vi "LV to ITX  Retrieve_SE mode.vi"(0 "File or Folder Path":path=path "G:/My Drive/ansom/Data/PPMS2/SA03008L.20190612/030_phi_90_Vamp_bg=30_IV_Testing/SA03008L.20190612.000014.itx", 5 "offset":i32, 7 "length":i32=1, 9 "index":T2={"A"=7, "B"=17, "C"=7, "D"=17, "E"=3, "N1"=2, "N2"=2, "N3"=3, "N4"=4, "A 1"=3, "A 2"=3, "C 1"=3, "C 2"=3, "E 2"=4}, 11 "stop":bool, 12 "file contains 2D data?":bool) -> (1 "Spherical coordinates":dbl[][](array[numeric]), 2 "long":cluster{i32[], dbl[]}(graph), 3 "G vs T":cluster{dbl[], dbl[]}(graph), 4 "A vs B":cluster{dbl[], dbl[]}[](graph), 6 "C vs D":cluster{dbl[], dbl[]}[](graph), 8 "E( = A)":dbl[][](graph)=[[1.0203117914485766e-05], [1.0451409415651452e-05], [1.0462825682376084e-05], [1.0239799983652948e-05], [9.906027918537444e-06], [9.668588795449023e-06], [9.554840000855235e-06], [9.476205145075346e-06], [9.320844077203883e-06], [9.198217260011043e-06], [9.317043476919502e-06], [9.695411083534662e-06], [1.0241945945024096e-05], [1.0795271186317606e-05], [1.1298338561231194e-05], [1.1790485816338598e-05], [1.2350446475265752e-05], [1.2919662467720538e-05], [1.3290994889745302e-05], [1.3411667855331416e-05], [1.330535085371591e-05], [1.3128995145360939e-05], [1.3030460580636378e-05], [1.2978894707939279e-05], [1.2876874119941293e-05], [1.2686944824355687e-05], [1.2580403309284722e-05], [1.2658289461507464e-05], [1.2907014184352959e-05], [1.3250891765203631e-05], [1.3571060207080296e-05], [1.38696075611843e-05], [1.4181218154607563e-05], [1.4550968177813745e-05], [1.4864220110273978e-05], [1.4963626262998592e-05], [1.483786218451115e-05], [1.454789392231275e-05], [1.4276013976759574e-05], [1.4093434987113507e-05], [1.394115331370823e-05], [1.3733942398008014e-05], [1.3498551722113728e-05], [1.3401834118376352e-05], [1.349625299977089e-05], [1.376633995345719e-05], [1.4099700190262174e-05], [1.439564212454811e-05], [1.4669263029595617e-05], [1.4993648567227242e-05], [1.5385015866889246e-05], [1.564851404848794e-05], [1.5665209617742956e-05], [1.5433872809106696e-05], [1.5053460371993616e-05], [1.4698589553022668e-05], [1.4387375425877016e-05], [1.4045380848753723e-05], [1.3602477208659444e-05], [1.3177214908981591e-05], [1.2924329669653593e-05], [1.2880547914446448e-05], [1.303231603971595e-05], [1.3248510272418485e-05], [1.3465963014008446e-05], [1.3681644430620408e-05], [1.3944747365597995e-05], [1.4215309953351151e-05], [1.431037322959714e-05], [1.4175945939035027e-05], [1.3817874591680678e-05], [1.3391248811154445e-05], [1.3062055548545288e-05], [1.2821830137320284e-05], [1.2576309609254846e-05], [1.2246815447133818e-05], [1.1922180751465795e-05], [1.1680853926483689e-05], [1.1589134778894471e-05], [1.1633830542786138e-05], [1.1704064673099467e-05], [1.1789993030575904e-05], [1.1926922111402669e-05], [1.215771870713351e-05], [1.2337490622128459e-05], [1.230294631547821e-05], [1.2038499839080447e-05], [1.1589020929183376e-05], [1.1155486186825546e-05], [1.0841489539352708e-05], [1.0586914588993357e-05], [1.0275705901404508e-05], [9.933726372538684e-06], [9.741201124246198e-06], [9.759761104382419e-06], [9.991224895934066e-06], [1.0316901386610578e-05], [1.0633212529286809e-05], [1.0935414635607847e-05], [1.127192689353356e-05], [1.168222121368369e-05], [1.1975070483694205e-05], [1.2017866014802864e-05], [1.182059565925867e-05], [1.1495227673116619e-05], [1.1221973090195048e-05], [1.102061719762733e-05], [1.0822809552516617e-05], [1.0531987977837665e-05], [1.0230877354511187e-05], [1.0096596104104945e-05], [1.0173052237292175e-05], [1.0421846888649233e-05], [1.0702637025924256e-05], [1.095426977171788e-05], [1.1200388597928466e-05], [1.1519306746724885e-05], [1.1877703630116518e-05], [1.2078276877349205e-05], [1.205320354878895e-05], [1.1810154186171108e-05], [1.1490160906859651e-05], [1.1235411490808346e-05], [1.1028963796796881e-05], [1.0777926144571402e-05], [1.0435400507185421e-05], [1.0169646968721249e-05], [1.010128110333465e-05], [1.0231121727379654e-05], [1.0469283566468044e-05], [1.0678876882796116e-05], [1.0845441918195888e-05], [1.1013496058458993e-05], [1.1250653310333545e-05], [1.1455840654342756e-05], [1.1487198402341834e-05], [1.1316332482261583e-05], [1.0965676444491303e-05], [1.0604440631932836e-05], [1.0327624088147793e-05], [1.0096830398805317e-05], [9.811227194429744e-06], [9.511062174305784e-06], [9.433820234221822e-06], [9.65222061750109e-06], [1.0092082217056494e-05], [1.0586760382445729e-05], [1.101426996619165e-05], [1.1384440045107256e-05], [1.1767057215702233e-05], [1.218251607479168e-05], [1.245159787228818e-05], [1.2481102402364999e-05], [1.2291430480708847e-05], [1.1986335326318682e-05], [1.1733869529760309e-05], [1.1548603391828037e-05], [1.13596762158455e-05], [1.1087736184421201e-05], [1.0839800019004791e-05], [1.076298217931536e-05], [1.087176289143856e-05], [1.1137984996962431e-05], [1.142759878667849e-05], [1.1672564147584565e-05], [1.189430562660553e-05], [1.2172128947557167e-05], [1.2459795985893852e-05], [1.2561260005336956e-05], [1.2424412782407364e-05], [1.2054150550705076e-05], [1.1589880038662732e-05], [1.1192416052986661e-05], [1.0863456381263106e-05], [1.051505112264767e-05], [1.0100597815099605e-05], [9.761572319705686e-06], [9.570513017820516e-06], [9.543303173198097e-06], [9.642325412517067e-06], [9.74774836365151e-06], [9.858949953493099e-06], [1.001903548052811e-05], [1.0256078261757475e-05], [1.0439598776211572e-05], [1.042242238004522e-05], [1.0183216760688765e-05], [9.769220768503082e-06], [9.367514440383908e-06], [9.053677195274377e-06], [8.770462725955242e-06], [8.43425116077764e-06], [8.081231920036751e-06], [7.879765327297044e-06], [7.889913212940979e-06], [8.1260164848618e-06], [8.447281143591908e-06], [8.695609460809765e-06], [8.902012120386912e-06], [9.171053878914142e-06], [9.519041688511399e-06], [9.760420847561693e-06], [9.77389276916549e-06], [9.538471022579816e-06], [9.15889899491702e-06], [8.826822020269094e-06], [8.565524931184424e-06], [8.289350815712172e-06], [7.8969407152003e-06], [7.459738307347468e-06], [7.128929719791946e-06], [6.99557875543524e-06], [7.060672622112839e-06], [7.158874263853444e-06], [7.221292908402365e-06], [7.283320382366653e-06], [7.412810700573441e-06], [7.557741133867653e-06], [7.536052902423093e-06], [7.301346793160131e-06], [6.860798082904608e-06], [6.352981206582646e-06], [5.915198962346519e-06], [5.513485928879271e-06], [5.042056071494383e-06], [4.47272121028262e-06], [3.990706674059657e-06], [3.711277759527869e-06], [3.648286875837285e-06], [3.736276427208576e-06], [3.846408121208589e-06], [3.94839189517527e-06], [4.081067676347965e-06], [4.321202984988554e-06], [4.539701763689317e-06], [4.560691591500203e-06], [4.362959065752805e-06], [4.00747885911292e-06], [3.684539738102325e-06], [3.457908230535235e-06], [3.256577421797549e-06], [2.982077739421097e-06], [2.677707243957301e-06], [2.527995181945928e-06], [2.563590932568395e-06], [2.757244015651364e-06], [3.004506737628388e-06], [3.216838705464376e-06], [3.411720821800805e-06], [3.65592557254819e-06], [3.966380574944244e-06], [4.154977498960543e-06], [4.109249917249561e-06], [3.827641578709879e-06], [3.415103581151261e-06], [3.060145017851194e-06], [2.788449265930315e-06], [2.531428415712389e-06], [2.223813484173366e-06], [1.961951236414797e-06], [1.873175358972362e-06], [1.978752723280979e-06], [2.235548987483699e-06], [2.487500911952594e-06], [2.680258099595024e-06], [2.857726048616139e-06], [3.101374069773001e-06], [3.360530904168342e-06], [3.439879860822285e-06], [3.285712948159889e-06], [2.920853244361546e-06], [2.517085401731428e-06], [2.227960344817152e-06], [2.019360394093301e-06], [1.790712123384404e-06], [1.490453406785682e-06], [1.314481541186986e-06], [1.436226320267349e-06], [1.830555611405548e-06], [2.347376474778584e-06], [2.83276224941652e-06], [3.273270977299852e-06], [3.720804122713015e-06], [4.225387814657854e-06], [4.643762651590139e-06], [4.818501878615677e-06], [4.74287964664764e-06], [4.484016645670352e-06], [4.23197417456386e-06], [4.052188441737428e-06], [3.878583078383493e-06], [3.6213318980411e-06], [3.320427547442246e-06], [3.144570932206806e-06], [3.145190133720137e-06], [3.342213788958479e-06], [3.643982192034937e-06], [3.950314414020666e-06], [4.273802952804333e-06], [4.665541321937886e-06], [5.116145221529651e-06], [5.437284100346412e-06], [5.532627391374035e-06], [5.39754437705853e-06], [5.128169611859323e-06], [4.896411012736348e-06], [4.725729377989505e-06], [4.570373201814337e-06], [4.358936049799571e-06], [4.191322167244521e-06], [4.217144518716558e-06], [4.445677705144123e-06], [4.827234705535528e-06], [5.222470576927392e-06], [5.582610826085262e-06], [5.934955025393205e-06], [6.340159015530785e-06], [6.731834383113837e-06], [6.909189589337826e-06], [6.827526507809335e-06], [6.512808994630573e-06], [6.124039292062173e-06], [5.789316724794161e-06], [5.474577386936262e-06], [5.115423045986515e-06], [4.695085634491939e-06], [4.371814745650077e-06], [4.238329052844964e-06], [4.29836974160633e-06], [4.47838263827086e-06], [4.6479008090333e-06], [4.787126253382991e-06], [4.932759271760401e-06], [5.15222285566227e-06], [5.314443835593722e-06], [5.249888099863707e-06], [4.955396042759312e-06], [4.49094662616732e-06], [4.032573470572639e-06], [3.652538610621264e-06], [3.289848568538427e-06], [2.862668862863305e-06], [2.386109658112519e-06], [1.980877493646386e-06], [1.723813276391883e-06], [1.666466791653346e-06], [1.708598627200872e-06], [1.750958161424472e-06], [1.803408641811402e-06], [1.924580144024447e-06], [2.131889646664636e-06], [2.23190345117017e-06], [2.101992507805945e-06], [1.746313784890978e-06], [1.282165699648718e-06], [9.008654645192786e-07], [6.245874645948886e-07], [3.603328178056157e-07], [1.2850462096549098e-08], [-2.9789678292108053e-07], [-3.9750583982440066e-07], [-2.555823624812689e-07], [7.11177067009668e-08], [4.2320008921387924e-07], [7.487434826133602e-07], [1.066972084992825e-06], [1.434819215080255e-06], [1.800878646893036e-06], [1.959611245457595e-06], [1.853971362801683e-06], [1.516878911187727e-06], [1.117968181486286e-06], [7.985815688218983e-07], [5.096106220425769e-07], [1.4977550826058187e-07], [-2.946925906959275e-07], [-6.300191196025e-07], [-7.439538241958556e-07], [-6.359796849249192e-07], [-3.886910298714256e-07], [-1.3897634048540907e-07], [9.549038154863474e-08], [3.508743558744578e-07], [6.84545669886253e-07], [9.691078084455289e-07], [1.045482439389716e-06], [8.974995121583454e-07], [5.802282921684991e-07], [2.7770754230560435e-07], [6.055233896067443e-08], [-1.217629251957688e-07], [-3.541677543525877e-07], [-5.957703521256667e-07], [-6.864721271250091e-07], [-5.986966950738157e-07], [-3.3156894730776936e-07], [-2.272892874096102e-09], [2.6674322548996125e-07], [4.88776088221634e-07], [7.363185836564282e-07], [1.030874484092974e-06], [1.204371480070388e-06], [1.161248106198924e-06], [8.881766431856405e-07], [4.88182629381204e-07], [1.6957924160034613e-07], [-3.531580448202741e-08], [-1.997832893026395e-07], [-4.102211628754495e-07], [-5.710429951959878e-07], [-4.961172001967793e-07], [-1.5114185155885382e-07], [3.744481859043512e-07], [9.191159334167871e-07], [1.430499110631943e-06], [1.919253087931085e-06], [2.445675439460715e-06], [2.988121323760386e-06], [3.368179636685896e-06], [3.48351381168019e-06], [3.322399885005343e-06], [3.07056014534199e-06], [2.903753127818985e-06], [2.79632673000765e-06], [2.637584615085359e-06], [2.383878891964776e-06], [2.203073403682545e-06], [2.206283438080234e-06], [2.405450646883647e-06], [2.716423840938837e-06], [2.997254703288021e-06], [3.241467706370339e-06], [3.511794372749976e-06], [3.868311613144331e-06], [4.15533629381371e-06], [4.203690567256924e-06], [4.006419102954573e-06], [3.618876334099121e-06], [3.236053706440711e-06], [2.934280935773519e-06], [2.643883040603065e-06], [2.264492261057744e-06], [1.851511625129745e-06], [1.612134189405098e-06], [1.583215981848726e-06], [1.729201609841909e-06], [1.944355531860828e-06], [2.13024641884391e-06], [2.283816621994958e-06], [2.477461369183668e-06], [2.728587070825201e-06], [2.847811614538933e-06], [2.751491004377477e-06], [2.449412680323661e-06], [2.044435640440341e-06], [1.721446280484857e-06], [1.497770951345898e-06], [1.293161644964387e-06], [1.010439134397641e-06], [7.454181515776826e-07], [6.603433933302327e-07], [7.876365575969897e-07], [1.086288853957634e-06], [1.410545885540973e-06], [1.70814523635708e-06], [2.018512138600734e-06], [2.421154123964878e-06], [2.851042034185028e-06], [3.09276890545274e-06], [3.091227660951088e-06], [2.872414028807718e-06], [2.596154472420182e-06], [2.405449023316103e-06], [2.274691555343845e-06], [2.10839650320063e-06], [1.8405205006478e-06], [1.588796015095602e-06], [1.460207742292944e-06], [1.516317184332083e-06], [1.712469405531179e-06], [1.901116704222114e-06], [2.050382524275238e-06], [2.208421297738088e-06], [2.444117414591197e-06], [2.646666143304353e-06], [2.668691134184238e-06], [2.474176299410271e-06], [2.105949975915483e-06], [1.765464179910295e-06], [1.526397172225546e-06], [1.32946264448765e-06], [1.088560883676088e-06], [8.227278560205486e-07], [6.864402022873568e-07], [7.299174399197152e-07], [9.672335319015463e-07], [1.30141719424543e-06], [1.6208334069415e-06], [1.913529408708613e-06], [2.220449994366263e-06], [2.563869674397319e-06], [2.788889776922702e-06], [2.791337202094483e-06], [2.559998735141068e-06], [2.201772202390378e-06], [1.899596496537296e-06], [1.672853353150462e-06], [1.444512065193071e-06], [1.128819750981524e-06], [8.408771228283138e-07], [7.573676174365871e-07], [9.045652354797287e-07], [1.222661558811304e-06], [1.572171244126944e-06], [1.892799603038695e-06], [2.194159561400824e-06], [2.55808916828674e-06], [2.929781042095453e-06], [3.105640547296532e-06], [3.04470953591822e-06], [2.77985109235159e-06], [2.477765739299556e-06], [2.263806449175554e-06], [2.089337566626353e-06], [1.857038796143934e-06], [1.531643873879591e-06], [1.287254079771486e-06], [1.228018805637217e-06], [1.359929120505531e-06], [1.626954183030257e-06], [1.899503641261853e-06], [2.149083748605454e-06], [2.424318021443189e-06], [2.771058966258793e-06], [3.03779347608129e-06], [3.070950972178974e-06], [2.862310179591683e-06], [2.472534202116903e-06], [2.08701427800541e-06], [1.773191081900734e-06], [1.475834316236762e-06], [1.107346170237545e-06], [7.217834878283793e-07], [5.400379788174451e-07], [6.384864116813995e-07], [9.723852081279428e-07], [1.394457283972456e-06], [1.800063013342451e-06], [2.192915874449245e-06], [2.620621076879388e-06], [3.089354051541878e-06], [3.43075078848014e-06], [3.535509574751654e-06], [3.385605436421143e-06], [3.09990916505182e-06], [2.854328439744856e-06], [2.649265060027011e-06], [2.427348435903839e-06], [2.130950149691371e-06], [1.874965331750264e-06], [1.800585266108255e-06], [1.922778247879644e-06], [2.209874864767858e-06], [2.517069382566403e-06], [2.777710512520955e-06], [3.025077599580109e-06], [3.344371123008913e-06], [3.670968838980564e-06], [3.805153528635349e-06], [3.719045967382481e-06], [3.4453056065883e-06], [3.121717158538113e-06], [2.867202531810868e-06], [2.666060001059221e-06], [2.446064840422678e-06], [2.182870825013239e-06], [2.031393827881757e-06], [2.064437873244976e-06], [2.274629467551607e-06], [2.572929205865769e-06], [2.828532692006165e-06], [3.046953258646045e-06], [3.282485366653173e-06], [3.602584247405248e-06], [3.880581588153572e-06], [3.958501824259167e-06], [3.812998042220891e-06], [3.500154747796919e-06], [3.220209945487412e-06], [3.033425363641895e-06], [2.860399775395278e-06], [2.61920739403021e-06], [2.370543731049188e-06], [2.287136477362237e-06], [2.413618613599854e-06], [2.747229106812454e-06], [3.159624133634061e-06], [3.537454804057392e-06], [3.886505667804312e-06], [4.274535372370747e-06], [4.730559591923031e-06], [5.063492431218344e-06], [5.157257415055617e-06], [5.005731444161624e-06], [4.719943355378965e-06], [4.487458764381221e-06], [4.335606809240858e-06], [4.196104531728331e-06], [3.967290069039871e-06], [3.728240982089026e-06], [3.615701464454324e-06], [3.683976766834997e-06], [3.934564789475532e-06], [4.228261965097601e-06], [4.502387528544013e-06], [4.779542484424882e-06], [5.117289121815712e-06], [5.449335107903793e-06], [5.58701981163888e-06], [5.487694869509108e-06], [5.176018183753834e-06], [4.819191726850881e-06], [4.546511619318568e-06], [4.300821328369082e-06], [3.99781338085952e-06], [3.62673275657825e-06], [3.355487904966211e-06], [3.274086263472789e-06], [3.372249691405775e-06], [3.582345894870657e-06], [3.784449257833265e-06], [3.961951546871228e-06], [4.174250564645887e-06], [4.484714742695696e-06], [4.74020001227765e-06], [4.763433680211768e-06], [4.540563757421029e-06], [4.145600443100241e-06], [3.768598878927397e-06], [3.471172633634845e-06], [3.191447933683471e-06], [2.837239398545553e-06], [2.463511586571342e-06], [2.270735427476304e-06], [2.294716771548237e-06], [2.504898408993516e-06], [2.794306132286138e-06], [3.068322981631204e-06], [3.339437133022253e-06], [3.666058584241702e-06], [4.035431693880267e-06], [4.263965590990658e-06], [4.269395932914149e-06], [4.052437885411495e-06], [3.725874661453007e-06], [3.469667161741944e-06], [3.285674775833183e-06], [3.093631254341317e-06], [2.835403027320849e-06], [2.661288889179454e-06], [2.71963741334409e-06], [2.983483155818505e-06], [3.371429906272921e-06], [3.735029322161288e-06], [4.042427897309145e-06], [4.339621134221055e-06], [4.698433044568193e-06], [5.051264781404729e-06], [5.207905217871494e-06], [5.134693036873634e-06], [4.855329659996543e-06], [4.522835077294536e-06], [4.264599217223204e-06], [4.0509608926548e-06], [3.797881884872371e-06], [3.480006869288144e-06], [3.307000859045598e-06], [3.434613753073963e-06], [3.830250793698165e-06], [4.335369985352999e-06], [4.806810326506096e-06], [5.243588355373231e-06], [5.698033177926932e-06], [6.234766917863396e-06], [6.720371003428815e-06], [6.998847270190049e-06], [7.044838590512829e-06], [6.902368063818684e-06], [6.7543073980886e-06], [6.672453056620447e-06], [6.606293176564262e-06], [6.474473183251771e-06], [6.31277456486036e-06], [6.286562865011889e-06], [6.452152101869052e-06], [6.800158649510438e-06], [7.203929198104126e-06], [7.562895282031667e-06], [7.888021258620359e-06], [8.239039473020091e-06], [8.626346460217915e-06], [8.877160655531826e-06], [8.885615965537383e-06], [8.625705887098092e-06], [8.212255192644841e-06], [7.839117684774636e-06], [7.518591920880371e-06], [7.184310792842499e-06], [6.77147094972243e-06], [6.390127428925089e-06], [6.171984080464439e-06], [6.146261082580145e-06], [6.297407503219818e-06], [6.472742201385194e-06], [6.608435299039607e-06], [6.756133415743732e-06], [7.015040583179219e-06], [7.330421268770488e-06], [7.478904508054431e-06], [7.374191363904208e-06], [7.027486025784916e-06], [6.611420746799494e-06], [6.267509783907579e-06], [5.953916635800534e-06], [5.576336008604536e-06], [5.122155234699542e-06], [4.758469980040258e-06], [4.568062244936127e-06], [4.569931379995312e-06], [4.705877665972491e-06], [4.839700599305497e-06], [4.959180515709513e-06], [5.131680469570321e-06], [5.410800967050358e-06], [5.63492714528286e-06], [5.642076968352041e-06], [5.408862788679098e-06], [4.970633871102984e-06], [4.502316899450866e-06], [4.084806234015227e-06], [3.682560840105224e-06], [3.217313239532915e-06], [2.721284890287605e-06], [2.344087479039076e-06], [2.153751782753977e-06], [2.175351195881462e-06], [2.298085624890723e-06], [2.430663518050305e-06], [2.589303835716231e-06], [2.846831744546804e-06], [3.214272130879574e-06], [3.486804163039535e-06], [3.532579461969519e-06], [3.333988553624396e-06], [3.019823207071486e-06], [2.786031977279591e-06], [2.631151717042815e-06], [2.475234004435696e-06], [2.254818436661476e-06], [2.067389328034075e-06], [2.065265302354666e-06], [2.278140295990367e-06], [2.629202221216723e-06], [2.968695184526776e-06], [3.259532435891047e-06], [3.543640533579852e-06], [3.906058832181727e-06], [4.290718558291195e-06], [4.502467158663368e-06], [4.476075533965759e-06], [4.229861183612979e-06], [3.942382521675467e-06], [3.747008475433462e-06], [3.592273249341639e-06], [3.391937829252852e-06], [3.137281734593259e-06], [2.987944717267124e-06], [3.027807941274348e-06], [3.263532901865624e-06], [3.615503595071192e-06], [3.957905863806523e-06], [4.300800643533351e-06], [4.696553717671453e-06], [5.180948646265811e-06], [5.615737328280651e-06], [5.839855918335066e-06], [5.800711875450168e-06], [5.558479023553354e-06], [5.336680797054845e-06], [5.21988745057688e-06], [5.15103716243991e-06], [5.026385613801526e-06], [4.873797724894876e-06], [4.880804007747624e-06], [5.121379320580249e-06], [5.576678638731952e-06], [6.098556023484293e-06], [6.559721282308638e-06], [6.955296106265266e-06], [7.365928969802948e-06], [7.810938752567327e-06], [8.101676528167088e-06], [8.145139783509919e-06], [7.942993550314822e-06], [7.615637396897443e-06], [7.35988897203179e-06], [7.182983777174719e-06], [6.990461325857249e-06], [6.696556979033658e-06], [6.444618668041451e-06], [6.453681360852392e-06], [6.737950822420221e-06], [7.177156498359516e-06], [7.599130181123634e-06], [7.952496337869775e-06], [8.284167250683303e-06], [8.690495760471493e-06], [9.111106186972426e-06], [9.332156225638901e-06], [9.2736603838523e-06], [8.96220755826182e-06], [8.587397056248976e-06], [8.278894636605606e-06], [7.986644499428533e-06], [7.637684408399613e-06], [7.229500925282656e-06], [6.925829067561365e-06], [6.828794333637653e-06], [6.94103030841548e-06], [7.171848740013674e-06], [7.386898356528749e-06], [7.577341225698792e-06], [7.81232012108494e-06], [8.15475265676454e-06], [8.472521406787539e-06], [8.600213080966157e-06], [8.48470330487799e-06], [8.19301084369165e-06], [7.93708548036568e-06], [7.758264647596739e-06], [7.567584777115642e-06], [7.287074336710751e-06], [6.960687275970134e-06], [6.761220358960227e-06], [6.767203885006181e-06], [6.969195375634884e-06], [7.240258254833264e-06], [7.487456137080917e-06], [7.728372524627712e-06], [8.039482515608698e-06], [8.419304704064716e-06], [8.664302138274093e-06], [8.673403381633778e-06], [8.436716570672818e-06], [8.063640320802858e-06], [7.76076936937861e-06], [7.543862969261696e-06], [7.317578956995582e-06], [7.020286638460658e-06], [6.769473801088076e-06], [6.68709995958075e-06], [6.806163262740344e-06], [7.100895939406111e-06], [7.418532425544495e-06], [7.703681796236309e-06], [7.98740889210498e-06], [8.344367457268606e-06], [8.709005327056942e-06], [8.880290049890652e-06], [8.813188228219227e-06], [8.529147961474942e-06], [8.179880513296687e-06], [7.90305562165154e-06], [7.665426242818122e-06], [7.382115236687453e-06], [7.041766769372422e-06], [6.770387569758972e-06], [6.653167006931177e-06], [6.749342094542293e-06], [6.988554084544051e-06], [7.218956246724879e-06], [7.427535333374542e-06], [7.674154601528099e-06], [8.01960467110565e-06], [8.31852983388635e-06], [8.397973851705224e-06], [8.230357832595724e-06], [7.88400898324451e-06], [7.570766259550508e-06], [7.375785735722442e-06], [7.224436058344639e-06], [7.006421995857997e-06], [6.767765131436185e-06], [6.693742407142669e-06], [6.846026938468187e-06], [7.208184862494163e-06], [7.64113228998166e-06], [8.031944377346954e-06], [8.394941884458741e-06], [8.810462288314407e-06], [9.299748755538284e-06], [9.68797921912603e-06], [9.862087269257206e-06], [9.798702016037122e-06], [9.603404704257265e-06], [9.45737877370418e-06], [9.374899761237335e-06], [9.275947991192528e-06], [9.075973698389197e-06], [8.873851266975431e-06], [8.84192920982261e-06], [9.04423972425257e-06], [9.428265483069637e-06], [9.842739872441383e-06], [1.0250459587834515e-05], [1.0670864121091388e-05], [1.1154740437351128e-05], [1.1643047519803226e-05], [1.194407029335555e-05], [1.1983635379958323e-05], [1.1772249489963287e-05], [1.1490701183782681e-05], [1.1282165766694284e-05], [1.1095319105273816e-05], [1.0829166236332026e-05], [1.0475252228196087e-05], [1.021231824758549e-05], [1.013525992086417e-05], [1.0238856471662613e-05], [1.0430006443808766e-05], [1.0579817605107706e-05], [1.0672328510062783e-05], [1.0744504311346475e-05], [1.0855920554635741e-05], [1.0893561240683626e-05], [1.0732040541983888e-05], [1.0349693173985373e-05], [9.788747955338097e-06], [9.241579865167468e-06], [8.785580398632577e-06], [8.353432333029214e-06], [7.840823960538163e-06], [7.324125562489893e-06], [7.038399495606467e-06], [7.037415844240456e-06], [7.247360377628e-06], [7.511151908699003e-06], [7.737354031391238e-06], [7.932403405355896e-06], [8.153054693434558e-06], [8.40861918703816e-06], [8.523440094833346e-06], [8.402177569283186e-06], [8.036979611164867e-06], [7.547971729404101e-06], [7.115440694614251e-06], [6.736895678269175e-06], [6.345466557530386e-06], [5.890701167924523e-06], [5.489673919212047e-06], [5.290647906631747e-06], [5.310604572752742e-06], [5.490037967956741e-06], [5.696370940500233e-06], [5.889571103946571e-06], [6.097304042971084e-06], [6.376594372352298e-06], [6.664925454130084e-06], [6.795732090399775e-06], [6.703851172636534e-06], [6.393464097212113e-06], [6.045076060215549e-06], [5.791937463036094e-06], [5.580004928172626e-06], [5.324738677265096e-06], [5.01871513869046e-06], [4.811173235535289e-06], [4.812329455660063e-06], [5.055930460798128e-06], [5.444943955843821e-06], [5.823087094253529e-06], [6.152640329807864e-06], [6.469965254096111e-06], [6.847124256698563e-06], [7.186722158616007e-06], [7.331624679070534e-06], [7.224832821690635e-06], [6.939610034634221e-06], [6.685188210675353e-06], [6.508378291869052e-06], [6.325543432368856e-06], [6.056690698828403e-06], [5.768019640905575e-06], [5.627262381495851e-06], [5.661690563434414e-06], [5.844740703087418e-06], [6.07576323035538e-06], [6.286380810953003e-06], [6.48825179187519e-06], [6.733351008989712e-06], [7.045495475931437e-06], [7.255448638692293e-06], [7.238806095125575e-06], [6.987938318159179e-06], [6.628087793238608e-06], [6.3293524473268e-06], [6.087415578487492e-06], [5.823789968964162e-06], [5.475504298562288e-06], [5.128244705968536e-06], [4.901291003358945e-06], [4.856033567696046e-06], [4.989659154838534e-06], [5.176340152059938e-06], [5.366665254389664e-06], [5.591727743067452e-06], [5.914959701940972e-06], [6.250725020137735e-06], [6.418271557670133e-06], [6.374111083155199e-06], [6.134879350964948e-06], [5.877929836894284e-06], [5.731024074296889e-06], [5.65181400245476e-06], [5.55329095570909e-06], [5.40242677655219e-06], [5.339070049735331e-06], [5.449502277163153e-06], [5.755602325365735e-06], [6.18630098982567e-06], [6.608330591914078e-06], [6.990598600161537e-06], [7.376315887741333e-06], [7.833246895039624e-06], [8.22049124733306e-06], [8.369043077882127e-06], [8.247816895823347e-06], [7.926112717320612e-06], [7.608622156430861e-06], [7.360609363450636e-06], [7.124113099849237e-06], [6.829034025833029e-06], [6.521567603303085e-06], [6.359412288860466e-06], [6.40771287265516e-06], [6.665486914495307e-06], [7.005154403139928e-06], [7.331218708535559e-06], [7.655783722217698e-06], [8.030634759533294e-06], [8.444132561013203e-06], [8.719777324025987e-06], [8.772486762521923e-06], [8.604136350036843e-06], [8.328138585040022e-06], [8.09799300031762e-06], [7.90518642188658e-06], [7.6870878825373e-06], [7.381821919296695e-06], [7.097881568228831e-06], [6.994675183947564e-06], [7.103593245191163e-06], [7.359714394615171e-06], [7.613266642150038e-06], [7.819992036693479e-06], [8.02767744962943e-06], [8.309494474340466e-06], [8.588453126097828e-06], [8.681941422892005e-06], [8.534044079599252e-06], [8.153272429500853e-06], [7.707659246118142e-06], [7.339016064353144e-06], [7.021251546818392e-06], [6.655443395305511e-06], [6.214829634113702e-06], [5.909286153681671e-06], [5.882720251233059e-06], [6.101932763411406e-06], [6.417243167310519e-06], [6.681184758790036e-06], [6.885304464171771e-06], [7.095740255791064e-06], [7.371843318841089e-06], [7.560050587361075e-06], [7.501669298307807e-06], [7.187579963038329e-06], [6.704741766374311e-06], [6.235850180316746e-06], [5.816391311641096e-06], [5.402330094299041e-06], [4.945983360290834e-06], [4.507585025759371e-06], [4.23915219258784e-06], [4.166777706197646e-06], [4.269934326566664e-06], [4.428750091869241e-06], [4.550143745781829e-06], [4.655606046277324e-06], [4.831989941404156e-06], [5.110882111935008e-06], [5.314921431388809e-06], [5.30942425585337e-06], [5.057597724762262e-06], [4.695937825153983e-06], [4.436679794266103e-06], [4.290223345298153e-06], [4.167438935380135e-06], [3.993345239305746e-06], [3.867406518169012e-06], [3.906801317552177e-06], [4.136817491845778e-06], [4.529801581162728e-06], [4.946552730613784e-06], [5.331801883974669e-06], [5.712590637137978e-06], [6.15481048114338e-06], [6.592308342593456e-06], [6.826718310992344e-06], [6.786423941771237e-06], [6.503160450850271e-06], [6.165250904156449e-06], [5.901694596001484e-06], [5.670805443741351e-06], [5.391512239043709e-06], [5.043950419241433e-06], [4.778755470680834e-06], [4.703885752495193e-06], [4.852978673041959e-06], [5.132034472256779e-06], [5.383614800538611e-06], [5.582431445748275e-06], [5.778230431409974e-06], [6.035983896607754e-06], [6.225519349909351e-06], [6.18753429192489e-06], [5.885997394214071e-06], [5.390538711638232e-06], [4.916062898532066e-06], [4.532450209241443e-06], [4.158852467825933e-06], [3.700816231249144e-06], [3.192393922287833e-06], [2.77173442943289e-06], [2.517366564966731e-06], [2.453933002694584e-06], [2.457427247477482e-06], [2.445329840496316e-06], [2.443798336842065e-06], [2.517502447479715e-06], [2.653463435805371e-06], [2.647121840629681e-06], [2.407431893072826e-06], [1.944918838748093e-06], [1.373900544471411e-06], [8.690071972701417e-07], [4.460043921971993e-07], [2.3994153027749404e-08], [-4.772078955812689e-07], [-9.296377263108274e-07], [-1.191004061239274e-06], [-1.258829336722795e-06], [-1.173707362944406e-06], [-1.067196910194635e-06], [-1.004980148273486e-06], [-9.509764854045485e-07], [-8.143432214688862e-07], [-6.716744628640852e-07], [-7.067849101043071e-07], [-9.494047204049328e-07], [-1.374243051121839e-06], [-1.826025758357163e-06], [-2.192528897153799e-06], [-2.506327601424659e-06], [-2.839377802118919e-06], [-3.208299688879845e-06], [-3.461748412095858e-06], [-3.516882533670836e-06], [-3.372442251141997e-06], [-3.124538407791523e-06], [-2.920973641594452e-06], [-2.763056374131571e-06], [-2.55936170587205e-06], [-2.254259879332272e-06], [-2.010730062395028e-06], [-1.975026277277693e-06], [-2.144855278320569e-06], [-2.441238613014749e-06], [-2.687695998678873e-06], [-2.845945852715577e-06], [-2.975560578566412e-06], [-3.172537206977433e-06], [-3.427483809330863e-06], [-3.570584644725091e-06], [-3.520032758012489e-06], [-3.28732054766788e-06], [-2.995438694136551e-06], [-2.718291245271894e-06], [-2.44149899304749e-06], [-2.109988266904257e-06], [-1.718588729845347e-06], [-1.450081144536925e-06], [-1.406960874423544e-06], [-1.595441015121595e-06], [-1.882654006289221e-06], [-2.072155179344364e-06], [-2.168651721292348e-06], [-2.263411199280198e-06], [-2.427839606953714e-06], [-2.53776457249619e-06], [-2.411223616426452e-06], [-2.025744930442276e-06], [-1.484038524859132e-06], [-9.556358586421368e-07], [-4.979904794857061e-07], [-8.145967180729153e-08], [3.7828523166056795e-07], [8.240880186866514e-07], [1.073114443325633e-06], [1.060884069606465e-06], [8.026762397548698e-07], [4.7472448327205143e-07], [1.9352779469350945e-07], [-7.331356057681563e-08], [-3.873362161763781e-07], [-7.68413076053395e-07], [-1.06570720098898e-06], [-1.182868935435797e-06], [-1.113724277538013e-06], [-9.448518353741357e-07], [-7.900336183186166e-07], [-6.49051435160385e-07], [-4.6752263685952496e-07], [-1.8907528916339287e-07], [4.4270885268319854e-08], [7.66022561950486e-08], [-1.1816752797395643e-07], [-4.783269771581619e-07], [-8.322573794351121e-07], [-1.136060026619281e-06], [-1.450256049337859e-06], [-1.862268245663191e-06], [-2.309338683840211e-06], [-2.602040475455354e-06], [-2.684479939844273e-06], [-2.570804153586183e-06], [-2.383992633473158e-06], [-2.225306636833003e-06], [-2.102356104424118e-06], [-1.944334054823846e-06], [-1.734306846824687e-06], [-1.659789284976614e-06], [-1.821827003817929e-06], [-2.218320028530671e-06], [-2.717045810437855e-06], [-3.141046767561048e-06], [-3.490658187099461e-06], [-3.852293640380142e-06], [-4.28495989717341e-06], [-4.651246996288762e-06], [-4.819126308315418e-06], [-4.785210524604372e-06], [-4.61048158104818e-06], [-4.430968947389278e-06], [-4.281625005564198e-06], [-4.130819573618683e-06], [-3.915144596412178e-06], [-3.705531286687277e-06], [-3.680887732625927e-06], [-3.889896007107419e-06], [-4.30741311251049e-06], [-4.758115486186734e-06], [-5.10784963465542e-06], [-5.386563780742694e-06], [-5.687526085896469e-06], [-6.066396755569145e-06], [-6.43210771436477e-06], [-6.699709822426458e-06], [-6.793378729876748e-06], [-6.760276730846019e-06], [-6.726691416958937e-06], [-6.702299282151128e-06], [-6.623092151521949e-06], [-6.453325048042292e-06], [-6.367292678785888e-06], [-6.50146902702056e-06], [-6.844601168815589e-06], [-7.322783223118941e-06], [-7.764215309376126e-06], [-8.121315829315704e-06], [-8.454712964447679e-06], [-8.84525435244587e-06], [-9.229732711027898e-06], [-9.429398376824442e-06], [-9.405471413971426e-06], [-9.200984492442941e-06], [-8.960052958110711e-06], [-8.773615580776288e-06], [-8.605941742068713e-06], [-8.374232577152442e-06], [-8.09698762460976e-06], [-7.98735140522612e-06], [-8.143630611421226e-06], [-8.543444546712995e-06], [-9.032276301894786e-06], [-9.428916198605932e-06], [-9.745615607847807e-06], [-1.0068957084819786e-05], [-1.0444554058779317e-05], [-1.072373885345171e-05], [-1.077131141698551e-05], [-1.0584313246494653e-05], [-1.024144322679202e-05], [-9.913623554324154e-06], [-9.637636478909363e-06], [-9.35356550425772e-06], [-8.994439617937459e-06], [-8.653253248106588e-06], [-8.527988538665782e-06], [-8.671379507189692e-06], [-9.048646145461648e-06], [-9.473165378204514e-06], [-9.814707926371303e-06], [-1.0127791469361429e-05], [-1.0511693357053846e-05], [-1.0974076878825284e-05], [-1.135196449125619e-05], [-1.156532236055504e-05], [-1.1613444456277262e-05], [-1.1579962504550232e-05], [-1.1580024732694497e-05], [-1.1611526698390805e-05], [-1.1617403050119093e-05], [-1.1532396257436424e-05], [-1.147363534048067e-05], [-1.1592350621810618e-05], [-1.193475550104526e-05], [-1.2443642725088017e-05], [-1.294100508666685e-05], [-1.3360879352525401e-05], [-1.3746586132316609e-05], [-1.4201922799127944e-05], [-1.468751794159799e-05], [-1.4996650317835732e-05], [-1.5052806932382978e-05], [-1.4914107774154547e-05], [-1.4737387147584988e-05], [-1.4611302903706154e-05], [-1.4524369520606566e-05], [-1.4405567199113703e-05], [-1.4250682745233905e-05], [-1.4241608945417716e-05], [-1.4482933516754928e-05], [-1.4998679428544107e-05], [-1.5658188497082744e-05], [-1.626797140288743e-05], [-1.6814567321499225e-05], [-1.7355912513609948e-05], [-1.7954972936228827e-05], [-1.850824636483608e-05], [-1.8893639847968466e-05], [-1.9090993917324113e-05], [-1.9140336886593993e-05], [-1.9173759827480337e-05], [-1.923397838223521e-05], [-1.930103668751253e-05], [-1.9317832336104656e-05], [-1.9374080581593506e-05], [-1.96604796557136e-05], [-2.020933446055844e-05], [-2.09869611066054e-05], [-2.1824211618654762e-05], [-2.2606728039144118e-05], [-2.3367047410002412e-05], [-2.418142706860687e-05], [-2.5068475124899732e-05], [-2.5858583682964438e-05], [-2.6461247778142584e-05], [-2.6883004928017213e-05], [-2.7217022733421174e-05], [-2.7581642178554886e-05], [-2.797491347471546e-05], [-2.8335614218775077e-05], [-2.8606675261307303e-05], [-2.893489956980329e-05], [-2.9476792454507668e-05], [-3.0249923907326548e-05], [-3.1167751851648724e-05], [-3.203872291991123e-05], [-3.2805374963481104e-05], [-3.353087400632633e-05], [-3.431665358413472e-05], [-3.511886434736196e-05], [-3.578072837592464e-05], [-3.6260431375286364e-05], [-3.658685520942688e-05], [-3.690067981728247e-05], [-3.728263053346312e-05], [-3.769488070680747e-05], [-3.805865293131319e-05], [-3.837587531013982e-05], [-3.8828935536899876e-05], [-3.9523517251129055e-05], [-4.046402456283516e-05], [-4.1507262420602644e-05], [-4.246637423585115e-05], [-4.3334632146558266e-05], [-4.41906960600533e-05], [-4.51092192806595e-05], [-4.6021093102493155e-05], [-4.682411436597088e-05], [-4.745548706253828e-05], [-4.7924072099689274e-05], [-4.8361027286061424e-05], [-4.8809983105873164e-05], [-4.9232930906689345e-05], [-4.9544942984936933e-05], [-4.981025510359012e-05], [-5.021260347060517e-05], [-5.080665778183088e-05], [-5.157839637097003e-05], [-5.2357802178820155e-05], [-5.301706234156894e-05], [-5.358954182190419e-05], [-5.4170661814348365e-05], [-5.478505568488254e-05], [-5.52658927660802e-05], [-5.5530974305003354e-05], [-5.558546364165458e-05], [-5.551664677272581e-05], [-5.543540959182117e-05], [-5.5348991134785185e-05], [-5.520577276801431e-05], [-5.4947948789861355e-05], [-5.475140764315094e-05], [-5.477824030959923e-05], [-5.5033890111200363e-05], [-5.5456020320439185e-05], [-5.5861324982787784e-05], [-5.618332176005347e-05], [-5.6475383919408245e-05], [-5.68270222588273e-05], [-5.7171087986153464e-05], [-5.733246005702452e-05], [-5.728528595330091e-05], [-5.706168471497476e-05], [-5.678558523975098e-05], [-5.6543263203548505e-05], [-5.6329735339227845e-05], [-5.607829661008891e-05], [-5.5780869846196426e-05], [-5.5609866951750836e-05], [-5.564318306534623e-05], [-5.5877244657115395e-05], [-5.61923546481866e-05], [-5.6444534626094375e-05], [-5.664612378053144e-05], [-5.686586795319028e-05], [-5.7178671900807656e-05], [-5.745706592910734e-05], [-5.756068812092536e-05], [-5.748185587864242e-05], [-5.725703527243406e-05], [-5.7012201378229246e-05], [-5.6804111705665504e-05], [-5.6601261940465014e-05], [-5.631127421733425e-05], [-5.600568697071896e-05], [-5.588028495244783e-05], [-5.598692380406992e-05], [-5.62985270785427e-05], [-5.6632958597791676e-05], [-5.684549031128803e-05], [-5.6944971293951195e-05], [-5.6995231360662805e-05], [-5.697861326713122e-05], [-5.6685803269321735e-05], [-5.601852831064893e-05], [-5.502767255506977e-05], [-5.385581651502898e-05], [-5.2647385267208055e-05], [-5.1409022211413896e-05], [-5.006903485971664e-05], [-4.857275157937879e-05], [-4.707554620511925e-05], [-4.5743873127595316e-05], [-4.4616375080548293e-05], [-4.3611897662023706e-05], [-4.253068683394778e-05], [-4.132024740380556e-05], [-4.0039587924876196e-05], [-3.8782601654700394e-05], [-3.7500174119446004e-05], [-3.603474990665464e-05], [-3.436038177872736e-05], [-3.251334147867329e-05], [-3.063074499042274e-05], [-2.879263632728844e-05], [-2.6963112019230662e-05], [-2.5054730746457307e-05], [-2.3086679208797324e-05], [-2.126986386364378e-05], [-1.9702813461349925e-05], [-1.8404080781284425e-05], [-1.725376625768268e-05], [-1.6056419178452623e-05], [-1.4797771058737505e-05], [-1.3593345022874012e-05], [-1.2532290990529612e-05], [-1.1453117316116989e-05], [-1.0200759766100853e-05], [-8.777830895484478e-06], [-7.244808350253156e-06], [-5.722970401973985e-06], [-4.251268975971968e-06], [-2.812021107139187e-06], [-1.332336698999324e-06], [1.1397597244044291e-07], [1.34409069355957e-06], [2.328935188743022e-06], [3.093156055443206e-06], [3.783855219333706e-06], [4.503676059589097e-06], [5.20369056568084e-06], [5.783436740944877e-06], [6.239126283680065e-06], [6.764270551567918e-06], [7.451086047708225e-06], [8.294698661890313e-06], [9.208575213360713e-06], [1.0066479833439703e-05], [1.0858177601322083e-05], [1.1657673146667409e-05], [1.2515306251514313e-05], [1.3256049303816463e-05], [1.3722405932277404e-05], [1.3904070334030362e-05], [1.3900665288035219e-05], [1.3925444962460862e-05], [1.402043473819316e-05], [1.411053872604738e-05], [1.4123823743274323e-05], [1.4089135594611057e-05], [1.411858956608697e-05], [1.4284433646690507e-05], [1.4619138156486194e-05], [1.5001668641152568e-05], [1.5349270121589984e-05], [1.5686283949846887e-05], [1.6082920453332494e-05], [1.6546713945447467e-05], [1.688968304216333e-05], [1.6980848319315798e-05], [1.680562676189309e-05], [1.652500703824317e-05], [1.631877486493524e-05], [1.6168030186057662e-05], [1.6001531242158836e-05], [1.5761382377547913e-05], [1.5558242483484595e-05], [1.5523136271776924e-05], [1.5668761166246087e-05], [1.592311096907001e-05], [1.614944973444803e-05], [1.6333349476611618e-05], [1.6523841577965787e-05], [1.6785101147255084e-05], [1.7033984860578196e-05], [1.7090156866324733e-05], [1.690415655009404e-05], [1.649880859307757e-05], [1.6047000188555447e-05], [1.5664609006145167e-05], [1.5313737903453964e-05], [1.4909058922041368e-05], [1.4434418519691083e-05], [1.406386819727024e-05], [1.3915206535076052e-05], [1.4016033673155967e-05], [1.4264948823413861e-05], [1.4505614931114552e-05], [1.4713856851707168e-05], [1.4955141293183572e-05], [1.528041199601289e-05], [1.5517838427916586e-05], [1.5521357892484003e-05], [1.529524663900651e-05], [1.4910061008113134e-05], [1.4544064179443117e-05], [1.426385198237609e-05], [1.401828237157675e-05], [1.371616459154899e-05], [1.3431467766935494e-05], [1.3336256963743628e-05], [1.344316408959772e-05], [1.3723026255192172e-05], [1.4045978695774857e-05], [1.4309666415058927e-05], [1.4539285649949806e-05], [1.4825931779211488e-05], [1.5164420828431951e-05], [1.534372518887931e-05], [1.5255940479685492e-05], [1.4923252748348703e-05], [1.4510760896020636e-05], [1.418667261611423e-05], [1.391175472702376e-05], [1.3597431452702008e-05], [1.3188412260286945e-05], [1.2828695074728082e-05], [1.271836632022873e-05], [1.2890092952449354e-05], [1.3239116812893695e-05], [1.359730037780101e-05], [1.3914185440514137e-05], [1.422816121679669e-05], [1.4614712663317624e-05], [1.4997868364477513e-05], [1.5196448907489736e-05], [1.5166280800432289e-05], [1.494330887171612e-05], [1.4694162346225285e-05], [1.4519336634164232e-05], [1.438500395109492e-05], [1.4220886126118853e-05], [1.400246500660648e-05], [1.3873714971734307e-05], [1.3928601704927876e-05], [1.418346216392764e-05], [1.4543764203529126e-05], [1.4878419867096056e-05], [1.5172782546654902e-05], [1.548650162643341e-05], [1.5885228364346098e-05], [1.621809959103842e-05], [1.6334080221855417e-05], [1.6225425227561592e-05], [1.597923682971488e-05], [1.5782532510223893e-05], [1.5669846571801158e-05], [1.55548677007755e-05], [1.533989971507564e-05], [1.5104555139138266e-05], [1.5035607093986188e-05], [1.5178961477181162e-05], [1.550997165473929e-05], [1.5893305473934724e-05], [1.6239732802993733e-05], [1.655713661151933e-05], [1.6920680768687754e-05], [1.7325887564430058e-05], [1.7566723164440566e-05], [1.7544822081840725e-05], [1.7258354053002133e-05], [1.684296812833716e-05], [1.6479320853199603e-05], [1.6183261860094898e-05], [1.5883924334873938e-05], [1.5514413729358703e-05], [1.5224542025217717e-05], [1.515136752711802e-05], [1.529604412279023e-05], [1.5611012649753868e-05], [1.5963724352106714e-05], [1.6303234479606253e-05], [1.664515881304228e-05], [1.7061076514425646e-05], [1.7457263399971348e-05], [1.7618445432539398e-05], [1.7499251436643773e-05], [1.7154312252957725e-05], [1.6772500170895296e-05], [1.6460956538121414e-05], [1.617692135633066e-05], [1.5843096742400316e-05], [1.545838916761821e-05], [1.5173698837152518e-05], [1.5066141294201702e-05], [1.517220169764422e-05], [1.5419541979321966e-05], [1.568317893583365e-05], [1.5959947262238678e-05], [1.6298610249064316e-05], [1.6723750793397724e-05], [1.706369701640293e-05], [1.7172699433791586e-05], [1.703953342157734e-05], [1.6758831792236632e-05], [1.653070106376597e-05], [1.6385899380832812e-05], [1.6257205539722077e-05], [1.607247603665993e-05], [1.5891410870005117e-05], [1.587695292596028e-05], [1.6082583380825648e-05], [1.6495863611893827e-05], [1.6990241148350215e-05], [1.746379079302107e-05], [1.7908089478581315e-05], [1.838370281477291e-05], [1.8874775125051258e-05], [1.9209618877404543e-05], [1.931684792477001e-05], [1.9191585181807914e-05], [1.895681295049498e-05], [1.8760940746719585e-05], [1.8594136370354237e-05], [1.8393056192160925e-05], [1.8109487168744597e-05], [1.7881499354204834e-05], [1.7833254805500897e-05], [1.7978748571764718e-05], [1.827688449917044e-05], [1.8574954580146708e-05], [1.8810086313080758e-05], [1.903314532314188e-05], [1.9331209255884442e-05], [1.9592323631931e-05], [1.9618644577624173e-05], [1.9388903518194257e-05], [1.8962029003832612e-05], [1.8533139144975754e-05], [1.8203277505088226e-05], [1.791295626503665e-05], [1.756532427019149e-05], [1.7157771697069085e-05], [1.6877915098757134e-05], [1.6815562403255315e-05], [1.6973538632493762e-05], [1.7258297473549154e-05], [1.7548689093593576e-05], [1.783462590346715e-05], [1.815842586339898e-05], [1.8554321105316614e-05], [1.8856958827330305e-05], [1.893167244014809e-05], [1.8775941997359865e-05], [1.8470775123871363e-05], [1.8202786045763364e-05], [1.7998636787179074e-05], [1.778682652892094e-05], [1.7496229114891403e-05], [1.7209854676829185e-05], [1.7137684293662118e-05], [1.7344719252504935e-05], [1.7762456800247985e-05], [1.8204274975002617e-05], [1.85708021222869e-05], [1.8881620216858534e-05], [1.920610293226094e-05], [1.9538301068829492e-05], [1.9699986734168202e-05], [1.9616443184447935e-05], [1.9293060262899512e-05], [1.885900130673253e-05], [1.849885549594225e-05], [1.821717221137117e-05], [1.7917355180568684e-05], [1.7526794704781475e-05], [1.7183598604776517e-05], [1.7044152467443644e-05], [1.715127458027255e-05], [1.7452720012757175e-05], [1.7778015030141446e-05], [1.8068739143702757e-05], [1.8368257101850536e-05], [1.8743670470187667e-05], [1.910566232949138e-05], [1.926853698745696e-05], [1.917834564535947e-05], [1.8873006996956397e-05], [1.8548782734233853e-05], [1.831851021492531e-05], [1.8121902223197002e-05], [1.7863392669223148e-05], [1.7551536329918433e-05], [1.7368363999403963e-05], [1.737859052620887e-05], [1.7551025802167452e-05], [1.7804524695885167e-05], [1.805360207027032e-05], [1.828248619527272e-05], [1.852625252459363e-05], [1.882933110169066e-05], [1.9041268180981853e-05], [1.9029518674385258e-05], [1.8775289849763527e-05], [1.8356782568889775e-05], [1.796190954019236e-05], [1.7631570542435827e-05], [1.731156281296382e-05], [1.6924582321768502e-05], [1.655431655666002e-05], [1.6382580015450982e-05], [1.642761459468412e-05], [1.664343346162662e-05], [1.689995740087557e-05], [1.7123953151359166e-05], [1.7336641844707467e-05], [1.7610082426734294e-05], [1.7933517873526823e-05], [1.810696073500512e-05], [1.804069298278951e-05], [1.7744377627598996e-05], [1.7360345666302073e-05], [1.7049784577313395e-05], [1.6797115464798315e-05], [1.652618471721008e-05], [1.616424874257291e-05], [1.5807769876837008e-05], [1.5566426821781382e-05], [1.5494660935208325e-05], [1.5601437642116725e-05], [1.5756002780750473e-05], [1.5901430228325e-05], [1.6089264725831355e-05], [1.6411059231466827e-05], [1.677546908156036e-05], [1.698027289453728e-05], [1.6959955643105256e-05], [1.6729781864495682e-05], [1.6463698310217663e-05], [1.6266083551894962e-05], [1.609471917788757e-05], [1.5878576793544123e-05], [1.5607964211015743e-05], [1.544458848109561e-05], [1.548372353888868e-05], [1.5734605594388485e-05], [1.6102927342112445e-05], [1.6443908017834715e-05], [1.672852698875536e-05], [1.7038812344284585e-05], [1.744152998314097e-05], [1.7763518092244364e-05], [1.785205592784938e-05], [1.768499142644416e-05], [1.733119795099225e-05], [1.699414131278803e-05], [1.6734782875739794e-05], [1.6490837269445642e-05], [1.6188981813444023e-05], [1.5898243467440737e-05], [1.577903108042604e-05], [1.585916258961155e-05], [1.6102297944852962e-05], [1.6384614204828068e-05], [1.6619092656251284e-05], [1.680286053495947e-05], [1.7025182678284772e-05], [1.7318550403226616e-05], [1.7494583454315537e-05], [1.743951674882691e-05], [1.7140835836150555e-05], [1.6730887485125185e-05], [1.6381043492634886e-05], [1.609759380135864e-05], [1.580520270212797e-05], [1.54170962444825e-05], [1.505626873735144e-05], [1.4883515450797021e-05], [1.4939516504856545e-05], [1.5174268941199278e-05], [1.5426567294454472e-05], [1.5627050811863954e-05], [1.5817223322036307e-05], [1.609777647106736e-05], [1.6374104272297193e-05], [1.6432132783259866e-05], [1.623005423437092e-05], [1.5811224703008995e-05], [1.5358475446324974e-05], [1.4998195428720583e-05], [1.469827868672722e-05], [1.4357255279345843e-05], [1.3964951740266222e-05], [1.373084178870309e-05], [1.3758491569078216e-05], [1.4002535137977533e-05], [1.4336529752135255e-05], [1.465067560887906e-05], [1.4945259574204514e-05], [1.528069602702153e-05], [1.5708903183272068e-05], [1.6065568441639197e-05], [1.620599754305449e-05], [1.6120018241604616e-05], [1.586602304717365e-05], [1.5604697873901722e-05], [1.538352210215115e-05], [1.515672009036373e-05], [1.4851375550017686e-05], [1.4544835568407947e-05], [1.4409299265583096e-05], [1.4480311705925545e-05], [1.47255130889753e-05], [1.499665314407254e-05], [1.5212724575491748e-05], [1.541722957532822e-05], [1.5695741523676187e-05], [1.604070193573629e-05], [1.625502338542104e-05], [1.6228348930830638e-05], [1.5961433781934054e-05], [1.560405961427602e-05], [1.5319932369448148e-05], [1.5100301095439872e-05], [1.4869750332086658e-05], [1.4563377822442678e-05], [1.4307483819757834e-05], [1.4249739631271035e-05], [1.4411443056961927e-05], [1.4712748150903531e-05], [1.50032188935589e-05], [1.5244217539777221e-05], [1.546884724716722e-05], [1.5744958232230607e-05], [1.598532848438834e-05], [1.600562241951822e-05], [1.5768029629703105e-05], [1.5334939813704513e-05], [1.4899005019038424e-05], [1.4553638095884326e-05], [1.4252201726382841e-05], [1.3908232796510204e-05], [1.351297224944636e-05], [1.3228719630969335e-05], [1.3124994852695238e-05], [1.3205572717774984e-05], [1.3379229730922525e-05], [1.351994627489216e-05], [1.3637576774623569e-05], [1.3797955453144574e-05], [1.401984720715713e-05], [1.414583110200447e-05], [1.4074291349838377e-05], [1.3795690162992504e-05], [1.337223940337073e-05], [1.2990859556816972e-05], [1.2694001349266286e-05], [1.2403378372336626e-05], [1.2025613377558874e-05], [1.1622569772577086e-05], [1.1327833601028811e-05], [1.1188473336708078e-05], [1.1242623663284236e-05], [1.1381355362041109e-05], [1.1506924792971587e-05], [1.1639492120529011e-05], [1.1855631882936477e-05], [1.210782076211018e-05], [1.2178509278947174e-05], [1.2011673207358948e-05], [1.1659441541059721e-05], [1.1266151206142507e-05], [1.0960923881380782e-05], [1.0719405632054354e-05], [1.0463908971159014e-05], [1.0129601090242275e-05], [9.86782131900118e-06], [9.827379891429907e-06], [1.0018883845310956e-05], [1.0390692177116233e-05], [1.0792131745409552e-05], [1.114986465783574e-05], [1.150663961759643e-05], [1.1952677953982558e-05], [1.2383477304470255e-05], [1.259286625174007e-05], [1.2521778125852729e-05], [1.2216693418179384e-05], [1.1889649208343389e-05], [1.1657458546016538e-05], [1.145965795148134e-05], [1.1201621297986146e-05], [1.0898989268371654e-05], [1.0736681787922446e-05], [1.078585933401745e-05], [1.1024793506329058e-05], [1.13542542952094e-05], [1.1658890183207327e-05], [1.1944824525022578e-05], [1.2290949640676648e-05], [1.2733218594220554e-05], [1.3092270962029362e-05], [1.3219944555308275e-05], [1.3110287414569852e-05], [1.2869469160821053e-05], [1.26885391740245e-05], [1.2589940885789969e-05], [1.249151296173048e-05], [1.2301697455420567e-05], [1.2091445797443448e-05], [1.2032519790657901e-05], [1.2188949090248259e-05], [1.255995885194832e-05], [1.2999763754539727e-05], [1.3404913038453874e-05], [1.379929367767939e-05], [1.4271753529739395e-05], [1.4801796082432547e-05], [1.5185728827605705e-05], [1.5334880566145244e-05], [1.5249169808452738e-05], [1.5066303241829843e-05], [1.4926392642118692e-05], [1.4795865870213951e-05], [1.462089298753415e-05], [1.4364781939916171e-05], [1.417727869852905e-05], [1.4232495278954056e-05], [1.4531238270832149e-05], [1.4959579704873091e-05], [1.5359476877059234e-05], [1.569266356676578e-05], [1.601682877260665e-05], [1.6414633748386637e-05], [1.678422637258304e-05], [1.694345461120064e-05], [1.6847957908344168e-05], [1.6531186454020878e-05], [1.6186974688171527e-05], [1.5929853160639584e-05], [1.5710974426090883e-05], [1.543553565705818e-05], [1.5090832623639638e-05], [1.4849689914380484e-05], [1.4812083338257219e-05], [1.4982038842287242e-05], [1.525796919539109e-05], [1.550945165672072e-05], [1.571678138702137e-05], [1.594058533043717e-05], [1.623573923878077e-05], [1.6457277257314406e-05], [1.646080034528867e-05], [1.621728928022015e-05], [1.5811096503145466e-05], [1.5440707347601683e-05], [1.5161456966804656e-05], [1.4908461054076843e-05], [1.4589952453101837e-05], [1.4252341407432132e-05], [1.4052693572799116e-05], [1.405820220719287e-05], [1.4252079871328891e-05], [1.4484957747919766e-05], [1.4656130498291376e-05], [1.4799471054216675e-05], [1.5012814988544714e-05], [1.528010932988113e-05], [1.5416555753190297e-05], [1.533336990942311e-05], [1.502984657580335e-05], [1.4658202088171737e-05], [1.4367583455843531e-05], [1.4109571756435352e-05], [1.3801850123664297e-05], [1.34066101675821e-05], [1.3054687551331031e-05], [1.2877987533860515e-05], [1.2908112723917993e-05], [1.3099266024429347e-05], [1.3329805135748422e-05], [1.3563601519915375e-05], [1.3822179815633094e-05], [1.4167555175052706e-05], [1.4494782556544853e-05], [1.460652008535624e-05], [1.4470418392856135e-05], [1.4146133668515353e-05], [1.3812713795542217e-05], [1.3557878640066333e-05], [1.3332213248377438e-05], [1.3062153336544928e-05], [1.2747009707907797e-05], [1.2509968099639297e-05], [1.2420959857474878e-05], [1.2537356994825586e-05], [1.2803185683125657e-05], [1.3095833650567017e-05], [1.3383353681202659e-05], [1.3712887035531382e-05], [1.4134031960650415e-05], [1.4485129570767477e-05], [1.4619492117046825e-05], [1.4520032682122913e-05], [1.4277448787521422e-05], [1.4080323651367223e-05], [1.396107816593502e-05], [1.3848798082364342e-05], [1.3652824548706134e-05], [1.3434254487286296e-05], [1.335391816233009e-05], [1.3471127617655986e-05], [1.3799911397786132e-05], [1.4223709704752634e-05], [1.4630991337687978e-05], [1.5011899427142152e-05], [1.545096156258362e-05], [1.5940007189051986e-05], [1.6279100655243503e-05], [1.637960393192634e-05], [1.6253410400314462e-05], [1.604345463771352e-05], [1.5898071209118093e-05], [1.5803879156082377e-05], [1.5686227061870915e-05], [1.5490788138924216e-05], [1.5354294223729025e-05], [1.5401522066086898e-05], [1.562867376569903e-05], [1.5953674689293744e-05], [1.6247569076878698e-05], [1.6502275850822093e-05], [1.6759907776586102e-05], [1.70664645506095e-05], [1.7332582896884287e-05], [1.741023340820019e-05], [1.726365156714191e-05], [1.6918617372296734e-05], [1.6547153095170146e-05], [1.6252980227367747e-05], [1.600432123778708e-05], [1.5714022834914565e-05], [1.536645893523311e-05], [1.5139498847017136e-05], [1.5141836413939582e-05], [1.5372663429099937e-05], [1.5711574295159004e-05], [1.6034744593455736e-05], [1.6343252999880454e-05], [1.6684972081312822e-05], [1.7091114272228252e-05], [1.7408229475361222e-05], [1.748677809505763e-05], [1.729831448393507e-05], [1.693680129982245e-05], [1.6591108988431626e-05], [1.6305892145530544e-05], [1.6020926034563266e-05], [1.562953889029583e-05], [1.5209850216327452e-05], [1.5006092942300278e-05], [1.5088711287249974e-05], [1.5375637148104433e-05], [1.5710168197066345e-05], [1.6023887696935973e-05], [1.633621857650097e-05], [1.6703541348254238e-05], [1.7086245539847025e-05], [1.7305438674712083e-05], [1.7309665340478807e-05], [1.7097065949415267e-05], [1.6776444304110332e-05], [1.6495695628181187e-05], [1.6242732863985817e-05], [1.5942645596805634e-05], [1.5551607568322378e-05], [1.5216186150569424e-05], [1.5073303832082367e-05], [1.5150790759881085e-05], [1.5404546344502117e-05], [1.5679166762616865e-05], [1.588459008881982e-05], [1.605437774469711e-05], [1.6296366114446896e-05], [1.6520275983354684e-05], [1.6534847953460887e-05], [1.6303267666730946e-05], [1.587055833390098e-05], [1.541649480257048e-05], [1.5045391361328337e-05], [1.4716233677716687e-05], [1.4346464602360635e-05], [1.395827755603539e-05], [1.3733265551716762e-05], [1.3740420208356257e-05], [1.3965387786255973e-05], [1.4299020165082598e-05], [1.4621594506664063e-05], [1.4932796465667902e-05], [1.5297160207141166e-05], [1.5738631973140124e-05], [1.6073027026669992e-05], [1.6167018638741076e-05], [1.6006325850163403e-05], [1.5680054534552332e-05], [1.5387595852749645e-05], [1.5163647062663941e-05], [1.4947282463811626e-05], [1.4668126802491151e-05], [1.438171870209571e-05], [1.4239186358959565e-05], [1.4297887741723659e-05], [1.4555804599507128e-05], [1.489370714501668e-05], [1.5209999854834479e-05], [1.5496884770818407e-05], [1.5816853323303903e-05], [1.615146052744146e-05], [1.6333525974233783e-05], [1.6292746446510267e-05], [1.604961212902166e-05], [1.575803659252903e-05], [1.5552691090088073e-05], [1.537566697267266e-05], [1.5123623222536933e-05], [1.4763114629776573e-05], [1.4421462789728673e-05], [1.4206118325486088e-05], [1.41590073322278e-05], [1.4243746221091115e-05], [1.433883351361289e-05], [1.4423977441522204e-05], [1.4551873740605627e-05], [1.47890233661317e-05], [1.5022570693774047e-05], [1.507526676601047e-05], [1.4894269652708548e-05], [1.449621551268247e-05], [1.4086710615905136e-05], [1.3789713987907603e-05], [1.3530471848631266e-05], [1.320166181399482e-05], [1.281881022802667e-05], [1.2570080039407714e-05], [1.2549743414549905e-05], [1.275263193204014e-05], [1.3070431552473942e-05], [1.3372869892852636e-05], [1.3620117553842693e-05], [1.3865255848509496e-05], [1.4169966200103845e-05], [1.4375789447240678e-05], [1.4352535947360882e-05], [1.409648017201831e-05], [1.3693340386991762e-05], [1.332787112033817e-05], [1.304561487644761e-05], [1.2785577696334131e-05], [1.2459674083621804e-05], [1.2139336538938602e-05], [1.1986305591187741e-05], [1.2026321630760766e-05], [1.2237299877831839e-05], [1.2518793731224008e-05], [1.279056064325593e-05], [1.3047094459395328e-05], [1.3363506851013705e-05], [1.3721296017680003e-05], [1.3913883751868719e-05], [1.3865450786586843e-05], [1.3608638461987529e-05], [1.3285780467760407e-05], [1.304762167167677e-05], [1.2878102766166168e-05], [1.269848883381341e-05], [1.2477482356196893e-05], [1.2346039629124877e-05], [1.2395866448600604e-05], [1.2642950366516907e-05], [1.3045903897388483e-05], [1.3446042305246994e-05], [1.3782050542316127e-05], [1.4106330606969869e-05], [1.4498817630373535e-05], [1.4869857959782323e-05], [1.5039496607221075e-05], [1.493739372174164e-05], [1.457710388613929e-05], [1.4145757353187369e-05], [1.3771573320222652e-05], [1.3435080003878147e-05], [1.3059843339237304e-05], [1.2653175078562846e-05], [1.2427260319859547e-05], [1.2495575004444683e-05], [1.281147698230303e-05], [1.3215899097485709e-05], [1.356246567670375e-05], [1.384071937777346e-05], [1.4123507745713618e-05], [1.4453108561599374e-05], [1.467180419763411e-05], [1.465981546108842e-05], [1.439834009535329e-05], [1.396274774094972e-05], [1.3543134223345296e-05], [1.3182995545791779e-05], [1.282350791879161e-05], [1.2402976213583424e-05], [1.201507380392556e-05], [1.1814296103600272e-05], [1.1836096789166112e-05], [1.2076141215238107e-05], [1.2393777593409726e-05], [1.2679143549999868e-05], [1.2959581001722879e-05], [1.3331243568101379e-05], [1.37533111311726e-05], [1.4005766273660908e-05], [1.4008380167202073e-05], [1.3761481046361242e-05], [1.3394373991721165e-05], [1.3082519078382114e-05], [1.2837176079072552e-05], [1.2577299766468597e-05], [1.2236625344424233e-05], [1.1953223677018107e-05], [1.1863466196077901e-05], [1.198050096587681e-05], [1.224712984890037e-05], [1.2533494426935635e-05], [1.2790182444836255e-05], [1.30566386713866e-05], [1.3407449735143829e-05], [1.3729951767474417e-05], [1.3839650424187614e-05], [1.3695856016676278e-05], [1.3345415509034565e-05], [1.2978731979064128e-05], [1.2684469003463e-05], [1.2408507259605167e-05], [1.2077969261800222e-05], [1.1715695800939766e-05], [1.1494556501591335e-05], [1.1473507841283281e-05], [1.1626678126170887e-05], [1.1866560793266924e-05], [1.2103858706163362e-05], [1.2339996064689047e-05], [1.2633865483964513e-05], [1.3017303775565921e-05], [1.330742276350848e-05], [1.3347813677236455e-05], [1.3124799185727358e-05], [1.2746802502681728e-05], [1.240887684586586e-05], [1.2139376297981079e-05], [1.1871251116008826e-05], [1.1517114602345373e-05], [1.1107199064010264e-05], [1.0778920603232481e-05], [1.0615039586135747e-05], [1.064340097963962e-05], [1.075531645369774e-05], [1.0867369136178985e-05], [1.1002521234184785e-05], [1.1238069627361565e-05], [1.1526340490400583e-05], [1.1653038024029704e-05], [1.1538116827136878e-05], [1.1199064583703464e-05], [1.0781610026671539e-05], [1.043405996501015e-05], [1.0119697437989108e-05], [9.747715357089713e-06], [9.293684978484134e-06], [8.934103316595763e-06], [8.794527267258078e-06], [8.874976357799646e-06], [9.12011456971441e-06], [9.38972888636345e-06], [9.635954751515362e-06], [9.901730406633756e-06], [1.0256361841227503e-05], [1.0591453275414255e-05], [1.0734395198913583e-05], [1.0653015024324325e-05], [1.0388986379758807e-05], [1.0125929506555288e-05], [9.95065272691937e-06], [9.804360954842187e-06], [9.594722886680921e-06], [9.336428006319844e-06], [9.215571164439007e-06], [9.290723643384585e-06], [9.546075524782364e-06], [9.895896565766293e-06], [1.0238454354828405e-05], [1.058867019380513e-05], [1.1005822769383501e-05], [1.150767997973763e-05], [1.1925635901660305e-05], [1.2126071867909224e-05], [1.2090471588612797e-05], [1.1907200353908402e-05], [1.1757632064967906e-05], [1.1671837939494583e-05], [1.1591479410316536e-05], [1.143694689095699e-05], [1.1269831428771994e-05], [1.124126366259789e-05], [1.1398937378405645e-05], [1.1730802052715057e-05], [1.2101919281567245e-05], [1.242745717621803e-05], [1.275500369720716e-05], [1.3190379035775244e-05], [1.3689935395678615e-05], [1.4037390651210099e-05], [1.4142085536546842e-05], [1.4005283565400679e-05], [1.3782720542962264e-05], [1.3631424354284837e-05], [1.3516349083932026e-05], [1.3344323404130796e-05], [1.3064393993936366e-05], [1.2844876153968495e-05], [1.2880357754220844e-05], [1.3191509101052876e-05], [1.3645774894309925e-05], [1.4061892479513102e-05], [1.440214573887559e-05], [1.4722802914466558e-05], [1.5115485996940762e-05], [1.550268020176897e-05], [1.570657393121205e-05], [1.566801489982928e-05], [1.5407015298102537e-05], [1.5109498841841007e-05], [1.4885213895367678e-05], [1.4664358844692019e-05], [1.4351608260559866e-05], [1.3972196513553053e-05], [1.3695011891292582e-05], [1.3606034822979478e-05], [1.3740952307349332e-05], [1.4008174352084425e-05], [1.4272579598894966e-05], [1.4524612174744851e-05], [1.4826479569030222e-05], [1.5199121435637785e-05], [1.5465348178397082e-05], [1.5499406159699886e-05], [1.52772103210063e-05], [1.4875981742185884e-05], [1.4492194060353827e-05], [1.4178556467900588e-05], [1.3880646101642747e-05], [1.352496134698449e-05], [1.3200557116711724e-05], [1.3042929028369806e-05], [1.3054553875854622e-05], [1.322908113860595e-05], [1.345249985511626e-05], [1.3633270885705617e-05], [1.378740694398623e-05], [1.3996041287563147e-05], [1.4245204907804839e-05], [1.435718514463492e-05], [1.4244469790444642e-05], [1.3910991129284788e-05], [1.3521223084710877e-05], [1.3234343758845636e-05], [1.3028408634242273e-05], [1.2810882578368993e-05], [1.2519470905079863e-05], [1.2288087426734334e-05], [1.2221333890027873e-05], [1.2329040373445925e-05], [1.257513335454784e-05], [1.2838441582443938e-05], [1.3079754450500774e-05], [1.3336995818657914e-05], [1.3672012724605868e-05], [1.3995979614154408e-05], [1.4152487399904576e-05], [1.4070674710797741e-05], [1.3752595291046939e-05], [1.3394965757998335e-05], [1.3119023736441995e-05], [1.288257758066815e-05], [1.2607415258317888e-05], [1.2275183305784112e-05], [1.2002957436706551e-05], [1.1901870216941609e-05], [1.2052837604836697e-05], [1.2373922862811369e-05], [1.2725268395095903e-05], [1.3071955363487625e-05], [1.3472720444867545e-05], [1.3968067821517188e-05], [1.4361938314276907e-05], [1.4509228898078139e-05], [1.4411366880491858e-05], [1.4166737851752824e-05], [1.3953380705410376e-05], [1.3785575183694125e-05], [1.3594235216339825e-05], [1.3312284682224201e-05], [1.302075049163835e-05], [1.2881270381473983e-05], [1.2942304598024198e-05], [1.318668078090307e-05], [1.3480188274563315e-05], [1.3740618022862066e-05], [1.3999000432341497e-05], [1.4327253566428847e-05], [1.4663210910980782e-05], [1.4813816596543845e-05], [1.4733577496283764e-05], [1.4427360188995282e-05], [1.4027749826961922e-05], [1.3700499583202787e-05], [1.3440800538572245e-05], [1.3167359675634943e-05], [1.2824081282807079e-05], [1.255662549428953e-05], [1.247494012603129e-05], [1.2580739623632583e-05], [1.2840981273177894e-05], [1.312292572948797e-05], [1.3373591405286142e-05], [1.3639668905490623e-05], [1.3997794920769625e-05], [1.4338612372276787e-05], [1.4478616690446433e-05], [1.4376447168444542e-05], [1.406469012599843e-05], [1.3729258567637082e-05], [1.3475390988927106e-05], [1.3254412615589495e-05], [1.2983522130158548e-05], [1.267820763622935e-05], [1.2493011770282791e-05], [1.248398363922502e-05], [1.2658294094307968e-05], [1.2941078368131056e-05], [1.3231554084034618e-05], [1.3517357172097023e-05], [1.3855746179641713e-05], [1.4282246018149822e-05], [1.461912915951853e-05], [1.4723241666775866e-05], [1.4576623928281488e-05], [1.4286297165004187e-05], [1.4066181391931139e-05], [1.3958859253159056e-05], [1.3881535444319144e-05], [1.3727678698561237e-05], [1.3575174845707965e-05], [1.3629683320838631e-05], [1.3943909492073762e-05], [1.444807400176148e-05], [1.4979678811445845e-05], [1.5432851297668823e-05], [1.5817212883753795e-05], [1.6237481651090774e-05], [1.6667008109983217e-05], [1.689469385793273e-05], [1.6861306130971918e-05], [1.660323551416216e-05], [1.627738320441142e-05], [1.6035151560723937e-05], [1.5838010156365698e-05], [1.558981519106848e-05], [1.5235339990811653e-05], [1.4916263046528974e-05], [1.4771164133527758e-05], [1.4827394399581081e-05], [1.5028200680119836e-05], [1.5218794686904256e-05], [1.53403504978672e-05], [1.5453798303518257e-05], [1.5640309978116142e-05], [1.5776907992513215e-05], [1.5700440710973434e-05], [1.539665628716548e-05], [1.489710553349513e-05], [1.4379757360876862e-05], [1.3961291483259452e-05], [1.3607994499762457e-05], [1.3223032862702087e-05], [1.2808523611056221e-05], [1.2532112725283956e-05], [1.2464548375089427e-05], [1.2612509633283844e-05], [1.2872604468710537e-05], [1.3124523197539775e-05], [1.3370964866684968e-05], [1.3680373751780775e-05], [1.4075357811308328e-05], [1.4351067101423046e-05], [1.4365854068547332e-05], [1.41327307849797e-05], [1.376870581321822e-05], [1.3455799168288345e-05], [1.3203168821220945e-05], [1.2935918394162637e-05], [1.258642945282157e-05], [1.2244104147973174e-05], [1.2060373915104194e-05], [1.2075795869588617e-05], [1.2270779287620338e-05], [1.2501151569471988e-05], [1.2686894143397115e-05], [1.2872374413804873e-05], [1.3144698164515417e-05], [1.3453643689482106e-05], [1.359870593717186e-05], [1.352582105610425e-05], [1.3271743843184017e-05], [1.2977874978910479e-05], [1.2780473760814187e-05], [1.2656307783391066e-05], [1.2507454791963335e-05], [1.2265244783418047e-05], [1.2040132564065666e-05], [1.1950317754446691e-05], [1.2047171428207438e-05], [1.2291984892039717e-05], [1.255878918903317e-05], [1.281311824785933e-05], [1.3103326408301461e-05], [1.3500052322292813e-05], [1.3893168225464474e-05], [1.4098270176696954e-05], [1.4057243106127296e-05], [1.381859044642029e-05], [1.3580037238136703e-05], [1.344735474459732e-05], [1.3380703931455165e-05], [1.3276752876166347e-05], [1.3116914944578913e-05], [1.30692941638584e-05], [1.3239450268501322e-05], [1.3621080027765885e-05], [1.4081300129519886e-05], [1.45141828989931e-05], [1.4932667544789758e-05], [1.539761447708412e-05], [1.5932767740986168e-05], [1.6355528677747e-05], [1.653026696220918e-05], [1.6449276485309654e-05], [1.6222924968947486e-05], [1.6035615365491194e-05], [1.5911836943727177e-05], [1.5802033511033997e-05], [1.5622989256764617e-05], [1.5444123635126828e-05], [1.544305496703508e-05], [1.5659762512024774e-05], [1.6035345854603076e-05], [1.6427029242298264e-05], [1.6776337258172307e-05], [1.711429202123924e-05], [1.7509420394215087e-05], [1.7911885497880992e-05], [1.8136993959182647e-05], [1.812233703371186e-05], [1.7874289092085996e-05], [1.7552234475018083e-05], [1.7304849743747594e-05], [1.709434936415987e-05], [1.682462546879593e-05], [1.6441797177161353e-05], [1.6110915386301813e-05], [1.597674729040627e-05], [1.6061144031740864e-05], [1.6296236462005678e-05], [1.6521137728426032e-05], [1.6688571315845896e-05], [1.6849086688950242e-05], [1.706577054368871e-05], [1.723395493004319e-05], [1.7190854023684907e-05], [1.6893306246049694e-05], [1.640751712403022e-05], [1.5943990055365646e-05], [1.5569499337552436e-05], [1.5214428688487364e-05], [1.4801973399342988e-05], [1.4355308914166129e-05], [1.4092171416892016e-05], [1.4126653937979416e-05], [1.4406968165691976e-05], [1.4781809276371705e-05], [1.5130185977515717e-05], [1.5438217223874122e-05], [1.577034848612662e-05], [1.6172669921420753e-05], [1.647601345756902e-05], [1.6542563752015053e-05], [1.637236641221073e-05], [1.607647107514394e-05], [1.582968081578582e-05], [1.563338268046079e-05], [1.5394282337393477e-05], [1.5048475634353377e-05], [1.4719375416870479e-05], [1.4577352222974707e-05], [1.4656324108218115e-05], [1.492028688216258e-05], [1.5211845731525799e-05], [1.543855740261186e-05], [1.5629580058022843e-05], [1.5877681588812385e-05], [1.6169201070589575e-05], [1.6322815074419254e-05], [1.6243436876684836e-05], [1.5932301867035406e-05], [1.5549036279966664e-05], [1.524099958459143e-05], [1.4989106313780492e-05], [1.4719378495660709e-05], [1.4378867742052099e-05], [1.4092292842489788e-05], [1.397584385297009e-05], [1.4047689530817077e-05], [1.4246890941907285e-05], [1.4433662684016598e-05], [1.45763759491657e-05], [1.4742304055792062e-05], [1.5006089299458814e-05], [1.5253215882814393e-05], [1.5308918134598822e-05], [1.512679725390057e-05], [1.4759065375631121e-05], [1.4407472147016304e-05], [1.414522852383408e-05], [1.391074316624162e-05], [1.3630640742683495e-05], [1.3325527668754515e-05], [1.316467242836264e-05], [1.3203902800324386e-05], [1.3426343328590399e-05], [1.3727720578436948e-05], [1.399715774510764e-05], [1.4251416378440344e-05], [1.4565540883417746e-05], [1.4945825359761927e-05], [1.5211241422005092e-05], [1.5253423795557723e-05], [1.5063237669970752e-05], [1.4739968715898735e-05], [1.446819686520028e-05], [1.4255610401413261e-05], [1.403266745657758e-05], [1.372502311613506e-05], [1.3390400237273681e-05], [1.318367385684198e-05], [1.3179472561699573e-05], [1.3364510056440581e-05], [1.3611955188888333e-05], [1.3858871950919623e-05], [1.4125205432906615e-05], [1.4468340703470662e-05], [1.482945428423405e-05], [1.5023602840992134e-05], [1.4986222200463028e-05], [1.4712459854440836e-05], [1.4349480444341565e-05], [1.4062579275537689e-05], [1.3829990324710162e-05], [1.3550574945562927e-05], [1.3183964653958983e-05], [1.2898644101841633e-05], [1.2830623727004027e-05], [1.299576578656341e-05], [1.3310445550304892e-05], [1.3611508365568668e-05], [1.3862756626380548e-05], [1.4124598525986394e-05], [1.4469573657989875e-05], [1.4798534304585838e-05], [1.4947853571510214e-05], [1.4866821242730922e-05], [1.4590250534720292e-05], [1.430554034780095e-05], [1.411018450374598e-05], [1.3957758641062074e-05], [1.3739491290426962e-05], [1.3445459296112932e-05], [1.325914042236078e-05], [1.3270477346493477e-05], [1.3474195713657593e-05], [1.3767948366493496e-05], [1.4038269971666784e-05], [1.4278688277129592e-05], [1.4553514984096848e-05], [1.4885922628500859e-05], [1.5089418560225952e-05], [1.5035341991069806e-05], [1.4729522320493105e-05], [1.4284048789083292e-05], [1.3894315195872797e-05], [1.3587111809704569e-05], [1.3280977463672477e-05], [1.2895568310790047e-05], [1.252807618421679e-05], [1.2333778534914969e-05], [1.233639729939717e-05], [1.2515120123800655e-05], [1.2743722302271112e-05], [1.2955560961180733e-05], [1.3182457307978107e-05], [1.348829892784507e-05], [1.381731929028348e-05], [1.3963136065791628e-05], [1.3846936515880674e-05], [1.3485703867457102e-05], [1.3037996442093253e-05], [1.266431766412486e-05], [1.2363489036047772e-05], [1.2072725725580551e-05], [1.1739884941880162e-05], [1.1510684352278436e-05], [1.15407099043401e-05], [1.1828961370198223e-05], [1.226795726145507e-05], [1.2707325183210768e-05], [1.310573672269998e-05], [1.350729803201214e-05], [1.3977246283816165e-05], [1.4406495998667438e-05], [1.4628546064855912e-05], [1.4610673259374812e-05], [1.4414547815362617e-05], [1.4240431606996144e-05], [1.4167986840458227e-05], [1.414642846523915e-05], [1.4101426326979754e-05], [1.401822791273574e-05], [1.404031602120524e-05], [1.4249715989769316e-05], [1.4638186242250855e-05], [1.5102994173727953e-05], [1.5534896296574975e-05], [1.59152935045224e-05], [1.6315681243152e-05], [1.678729809923617e-05], [1.7154999067391366e-05], [1.727245605562279e-05], [1.7121542128847572e-05], [1.6821335872188796e-05], [1.6584417508162956e-05], [1.6429235629912017e-05], [1.626381504022034e-05], [1.6014865491183458e-05], [1.5785692640923273e-05], [1.573765948770935e-05], [1.588820278344821e-05], [1.6187462652164212e-05], [1.6489969399084454e-05], [1.6716241653321113e-05], [1.6904598268401463e-05], [1.714846948668637e-05], [1.7414542920240364e-05], [1.7511073282369002e-05], [1.7364255472285388e-05], [1.6994088324339914e-05], [1.656223477799446e-05], [1.6216275817671493e-05], [1.5929952216326374e-05], [1.562035857679948e-05], [1.5231776132262531e-05], [1.4898421202602072e-05], [1.4748374082478684e-05], [1.4798987770335345e-05], [1.499073816744852e-05], [1.5192596536185059e-05], [1.5354009351377565e-05], [1.5517584482265803e-05], [1.5769698926434212e-05], [1.600133844185714e-05], [1.6029181662052326e-05], [1.5816213420679444e-05], [1.541761619718636e-05], [1.502731625354894e-05], [1.4737998370749626e-05], [1.4492704386044173e-05], [1.4204216915065542e-05], [1.3878687455444555e-05], [1.3640046129244882e-05], [1.3542668570170751e-05], [1.3613301992311637e-05], [1.3763926279084539e-05], [1.3884785680236355e-05], [1.400327459018405e-05], [1.4221710297158916e-05], [1.4560577002186693e-05], [1.4816368645330413e-05], [1.4852661533143729e-05], [1.4657390238912811e-05], [1.4330147385770699e-05], [1.4067007441205754e-05], [1.3893108291378242e-05], [1.3717723647996104e-05], [1.3450831136011257e-05], [1.3197586597843353e-05], [1.314361166318737e-05], [1.3317252756031614e-05], [1.3677169084753853e-05], [1.409198961534545e-05], [1.4477558897715503e-05], [1.4860868399384432e-05], [1.531705024499937e-05], [1.5785086750350087e-05], [1.6072494553869616e-05], [1.6126558639237043e-05], [1.5972042739751756e-05], [1.5760989335251145e-05], [1.5638211559988967e-05], [1.559111227903386e-05], [1.5535728886855924e-05], [1.539195698634976e-05], [1.5293139158515488e-05], [1.5367307315392288e-05], [1.5613468845536082e-05], [1.5958057499739333e-05], [1.6260384748783408e-05], [1.6490707871855102e-05], [1.672201325454372e-05], [1.7037851366860684e-05], [1.732393036599217e-05], [1.7398509696298844e-05], [1.721077201919406e-05], [1.6810902236319798e-05], [1.6405519234042853e-05], [1.6084692884340137e-05], [1.5780872455504395e-05], [1.540241449957088e-05], [1.4978783017350626e-05], [1.4693588091334184e-05], [1.4623351525538662e-05], [1.4790410830888815e-05], [1.5102057571967046e-05], [1.540137425778209e-05], [1.5654054753468167e-05], [1.593600786011744e-05], [1.629335844943609e-05], [1.6549756846393615e-05], [1.656228428088658e-05], [1.631772541113863e-05], [1.59310632127711e-05], [1.5600953847851506e-05], [1.5349904583568913e-05], [1.5106081204278572e-05], [1.479521848916646e-05], [1.4519311586052554e-05], [1.4476144884032507e-05], [1.4690715195521358e-05], [1.5075839535849021e-05], [1.5482727442688062e-05], [1.5827685170911652e-05], [1.611916191955137e-05], [1.64489219946971e-05], [1.679348293536779e-05], [1.6965527579206008e-05], [1.6899765227297515e-05], [1.661534606572882e-05], [1.627687810292188e-05], [1.6037136604237154e-05], [1.5869509546063736e-05], [1.5686448096978795e-05], [1.5422755852223563e-05], [1.5204090363667567e-05], [1.5151522877391342e-05], [1.5282682205116007e-05], [1.5535582839276648e-05], [1.5777551388144146e-05], [1.5978866713195457e-05], [1.6203691461159676e-05], [1.6524782157638495e-05], [1.6815647235944657e-05], [1.6887979439980315e-05], [1.6699616299238345e-05], [1.6316454680672362e-05], [1.5931575205341186e-05], [1.561940549671919e-05], [1.533135360478097e-05], [1.4998152983879448e-05], [1.4639181994907698e-05], [1.4400473101555566e-05], [1.4349554531193736e-05], [1.450619307303936e-05], [1.4760590181901054e-05], [1.4985346644726342e-05], [1.5181777207112603e-05], [1.5417430781455197e-05], [1.572280399573965e-05], [1.5932162176425995e-05], [1.5917088030068864e-05], [1.5658437445751966e-05], [1.5258417142388377e-05], [1.4906269732230025e-05], [1.4623507535472124e-05], [1.4330122017588753e-05], [1.3957149699714642e-05], [1.3623521073499209e-05], [1.349249968052347e-05], [1.3583856737149044e-05], [1.3856331070596274e-05], [1.415246893179716e-05], [1.4379788002418877e-05], [1.4587439833430134e-05], [1.4892621784188354e-05], [1.524881580109761e-05], [1.5424556543518312e-05], [1.5335556180171188e-05], [1.501263757388796e-05], [1.4615548423543437e-05], [1.4280727224622124e-05], [1.3984664968990338e-05], [1.366118962143892e-05], [1.328963791780297e-05], [1.2990636147716895e-05], [1.2836887366053474e-05], [1.2870503979571462e-05], [1.3084509514162634e-05], [1.3353819788790051e-05], [1.3615485905191467e-05], [1.3902929505390637e-05], [1.429022265660358e-05], [1.4659898649700796e-05], [1.4846639223470435e-05], [1.4811589281675762e-05], [1.4587983751275764e-05], [1.4374179749120937e-05], [1.4269937544315642e-05], [1.4221001160351966e-05], [1.4131115849210795e-05], [1.4017101411674632e-05], [1.4050705596946564e-05], [1.4277618864720926e-05], [1.4691302739779794e-05], [1.5212882740250313e-05], [1.5719462698902762e-05], [1.6192490737055782e-05], [1.6722383426373832e-05], [1.7343328948644582e-05], [1.7858167687803826e-05], [1.8134767270308374e-05], [1.8154055332232797e-05], [1.8004039988347783e-05], [1.7861113638451145e-05], [1.7754486959107328e-05], [1.7640593575338198e-05], [1.7462576077117077e-05], [1.7300810937385785e-05], [1.7308693318476738e-05], [1.7535550960754942e-05], [1.795571188952411e-05], [1.843381036984172e-05], [1.8874082887141516e-05], [1.9269321244239493e-05], [1.9687102689203003e-05], [2.010085503263589e-05], [2.033101087377135e-05], [2.029441237924691e-05], [2.000924880937927e-05], [1.9650437396589854e-05], [1.935109366732078e-05], [1.9062563507987117e-05], [1.8708843039985336e-05], [1.8275123739453217e-05], [1.792821435114401e-05], [1.7787578252157072e-05], [1.7858893707124236e-05], [1.807728931320474e-05], [1.8307034893751865e-05], [1.850676759650253e-05], [1.8717351212811967e-05], [1.8998071310249748e-05], [1.923221787191556e-05], [1.924647816810917e-05], [1.9007784870199143e-05], [1.8587514052624886e-05], [1.8183531658363878e-05], [1.7878777977008658e-05], [1.761778429456651e-05], [1.7291798311823047e-05], [1.691747799497573e-05], [1.672726910203886e-05], [1.6817240069081827e-05], [1.7131676342645442e-05], [1.7526908077548385e-05], [1.7874380638794923e-05], [1.81669414673539e-05], [1.848080300067523e-05], [1.8853388137447215e-05], [1.912284826352131e-05], [1.9169868512417135e-05], [1.8977678487506715e-05], [1.8647648865328004e-05], [1.8358343735130226e-05], [1.813328390431186e-05], [1.7921846301400666e-05], [1.764706958131821e-05], [1.7396680343192743e-05], [1.7334151366848404e-05], [1.7483169110904108e-05], [1.7817918975414482e-05], [1.8208310796756084e-05], [1.8560888280442107e-05], [1.8898937254912896e-05], [1.9310805364014996e-05], [1.9762342339293847e-05], [2.006599158831854e-05], [2.0125630515676716e-05], [1.9926096989126134e-05], [1.9631241319984495e-05], [1.938991829104e-05], [1.9171387262417375e-05], [1.8919016534561697e-05], [1.860704311211258e-05], [1.83681372749472e-05], [1.831639739072786e-05], [1.8467551021982567e-05], [1.876040033692301e-05], [1.9060068259582032e-05], [1.93087888766871e-05], [1.9553436725568646e-05], [1.9891011379076267e-05], [2.0215541911730603e-05], [2.0344825272138517e-05], [2.0219439925940936e-05], [1.989142701806474e-05], [1.9573412640188803e-05], [1.934202996716211e-05], [1.9126899050051145e-05], [1.884205268352124e-05], [1.8511873545713598e-05], [1.8308734754241056e-05], [1.8291797161453338e-05], [1.8455870028097447e-05], [1.870841222237378e-05]], 10 "N":cluster{"N1":dbl, "N2":dbl, "N3":dbl, "N4":dbl}={"N1"=0.0, "N2"=0.0, "N3"=0.0, "N4"=0.042391166609344784} {"N4" format="%#_6p"; "N3" format="%#_6p"; "N2" format="%#_6p"; "N1" format="%#_6p"}, 13 "Index, Wavenames":string[][](table)=[["0", "'time.SA03008L.20190612.000014'\n"], ["1", "'temp.SA03008L.20190612.000014'\n"], ["2", "'B.SA03008L.20190612.000014'\n"], ["3", "'Brate.SA03008L.20190612.000014'\n"], ["4", "'Lockin1.SA03008L.20190612.000014'\n"], ["5", "'Lockin2.SA03008L.20190612.000014'\n"], ["6", "'Lockin3.SA03008L.20190612.000014'\n"], ["7", "'Lockin4.SA03008L.20190612.000014'\n"], ["8", "'Lockin5.SA03008L.20190612.000014'\n"], ["9", "'Lockin6.SA03008L.20190612.000014'\n"], ["10", "'AO1.SA03008L.20190612.000014'\n"], ["11", "'AO2.SA03008L.20190612.000014'\n"], ["12", "'AO3.SA03008L.20190612.000014'\n"], ["13", "'AO4.SA03008L.20190612.000014'\n"], ["14", "'AO5.SA03008L.20190612.000014'\n"], ["15", "'AO6.SA03008L.20190612.000014'\n"], ["16", "'AO7.SA03008L.20190612.000014'\n"], ["17", "'AO8.SA03008L.20190612.000014'\n"], ["", ""]], 14 "Comments":string="IGOR\nX// Date: 6/13/2019 4:54 PM\nX// Device:\nX//     Device: SA03008L.20190612\nX//     Instrument: PPMS2\nX//     Computer: LLABWORKSTATION\nX//     User: Phil John\nX//     Description: SketchSET\nX// \nX// Wiring:\nX//     Electrode 1: Lockin 1, V1+, KH 1: SE+ (-gnd), 1x, Open\nX//     Electrode 2: Lockin 2, Vsg, KH 2: Differential, 10x, 50k Ohms\nX//     Electrode 3: Lockin 3, V1-, KH 3: SE+ (-gnd), 10x, Open\nX//     Electrode 4: Lockin 4, I-, KH 4: Differential, 10x, 50k Ohms\nX//     Electrode 5: Lockin 5, Vsg, KH 5: Differential, 10x, 50k Ohms\nX//     Electrode 27: Lockin 7, Vbg, KH 7: Differential, 10x, 50k Ohms\nX//     Electrode 28: Lockin 8, I+, KH 8: Differential, 10x, 50k Ohms\nX//     Electrode 1: Vbg\nX// \nX// Experiment: \nX//     bg 0.5*20 = 16V\nX//     ch8 250m\nX//     vsg2 0 to 500m inc5m\nX//     bg = 16\nX//     \nX//     *swapped resistors, Vsg2 now has 10M resistor\nX// \nX// Lockin: \nX//     AO 1: amp = 0.000 mV, DC = 0.000 mV, f = 0.30 Hz, phi = 0.00°, Triangle\nX//     AO 2: amp = 0.000 mV, DC = 0.000 mV, f = 0.30 Hz, phi = 0.00°, Triangle\nX//     AO 3: amp = 0.000 mV, DC = 0.000 mV, f = 0.30 Hz, phi = 0.00°, Triangle\nX//     AO 4: amp = 0.000 mV, DC = 0.000 mV, f = 0.30 Hz, phi = 0.00°, Triangle\nX//     AO 5: amp = 0.000 mV, DC = 0.000 mV, f = 0.30 Hz, phi = 0.00°, Triangle\nX//     AO 6: amp = 0.000 mV, DC = 0.000 mV, f = 0.30 Hz, phi = 0.00°, Triangle\nX//     AO 7: amp = 0.000 mV, DC = 0.000 mV, f = 0.30 Hz, phi = 0.00°, Triangle\nX//     AO 8: amp = 200.005 mV, DC = 0.000 mV, f = 0.30 Hz, phi = 90.00°, Triangle\nX// \nX//     Lockin 1: f = 0.30 Hz, phi = 90.00° \nX// \nX//     TC = 300.00 ms, order = 2\nX// \nX//     Fs = 1000.00 S/s, N = 3330 S\nX// \n\n\n\n\n\n\n\n\n\n\n\n\n\n\n\n\n\n\n\n\n\n\n\n\n\n\n\n\n\n\n\n\n\n\n\n\n\n\nX \nX Display/R 'time.SA03008L.20190612.000014'\nX AppendToGraph 'temp.SA03008L.20190612.000014'\nX AppendToGraph 'B.SA03008L.20190612.000014'\nX AppendToGraph 'Brate.SA03008L.20190612.000014'\nX AppendToGraph 'Lockin1.SA03008L.20190612.000014'\nX AppendToGraph 'Lockin2.SA03008L.20190612.000014'\nX AppendToGraph 'Lockin3.SA03008L.20190612.000014'\nX AppendToGraph 'Lockin4.SA03008L.20190612.000014'\nX AppendToGraph 'Lockin5.SA03008L.20190612.000014'\nX AppendToGraph 'Lockin6.SA03008L.20190612.000014'\nX AppendToGraph 'AO1.SA03008L.20190612.000014'\nX AppendToGraph 'AO2.SA03008L.20190612.000014'\nX AppendToGraph 'AO3.SA03008L.20190612.000014'\nX AppendToGraph 'AO4.SA03008L.20190612.000014'\nX AppendToGraph 'AO5.SA03008L.20190612.000014'\nX AppendToGraph 'AO6.SA03008L.20190612.000014'\nX AppendToGraph 'AO7.SA03008L.20190612.000014'\nX AppendToGraph 'AO8.SA03008L.20190612.000014'\nX Label bottom \"x label\"\nX Label left \"y label\"\nX ModifyGraph rgb('time.SA03008L.20190612.000014')=(65280,0,0)\nX ModifyGraph rgb('temp.SA03008L.20190612.000014')=(65280,11565,0)\nX ModifyGraph rgb('B.SA03008L.20190612.000014')=(65280,23130,0)\nX ModifyGraph rgb('Brate.SA03008L.20190612.000014')=(65280,34680,0)\nX ModifyGraph rgb('Lockin1.SA03008L.20190612.000014')=(65280,46155,0)\nX ModifyGraph rgb('Lockin2.SA03008L.20190612.000014')=(65280,57630,0)\nX ModifyGraph rgb('Lockin3.SA03008L.20190612.000014')=(57600,65280,0)\nX ModifyGraph rgb('Lockin4.SA03008L.20190612.000014')=(34560,65280,0)\nX ModifyGraph rgb('Lockin5.SA03008L.20190612.000014')=(11520,65280,0)\nX ModifyGraph rgb('Lockin6.SA03008L.20190612.000014')=(0,53760,11520)\nX ModifyGraph rgb('AO1.SA03008L.20190612.000014')=(0,30720,34560)\nX ModifyGraph rgb('AO2.SA03008L.20190612.000014')=(0,7680,57600)\nX ModifyGraph rgb('AO3.SA03008L.20190612.000014')=(7710,0,65280)\nX ModifyGraph rgb('AO4.SA03008L.20190612.000014')=(19275,0,65280)\nX ModifyGraph rgb('AO5.SA03008L.20190612.000014')=(30840,0,65280)\nX ModifyGraph rgb('AO6.SA03008L.20190612.000014')=(42330,0,65280)\nX ModifyGraph rgb('AO7.SA03008L.20190612.000014')=(53805,0,65280)\nX ModifyGraph rgb('AO8.SA03008L.20190612.000014')=(65280,0,65280)\nX Legend/C/N=text0/J \"\\\\s('time.SA03008L.20190612.000014') time\\r\\\\s('temp.SA03008L.20190612.000014') temp\\r\\\\s('B.SA03008L.20190612.000014') B\\r\\\\s('Brate.SA03008L.20190612.000014') Brate\\r\\\\s('Lockin1.SA03008L.20190612.000014') Lockin1\\r\\\\s('Lockin2.SA03008L.20190612.000014') Lockin2\\r\\\\s('Lockin3.SA03008L.20190612.000014') Lockin3\\r\\\\s('Lockin4.SA03008L.20190612.000014') Lockin4\\r\\\\s('Lockin5.SA03008L.20190612.000014') Lockin5\\r\\\\s('Lockin6.SA03008L.20190612.000014') Lockin6\\r\\\\s('AO1.SA03008L.20190612.000014') AO1\\r\\\\s('AO2.SA03008L.20190612.000014') AO2\\r\\\\s('AO3.SA03008L.20190612.000014') AO3\\r\\\\s('AO4.SA03008L.20190612.000014') AO4\\r\\\\s('AO5.SA03008L.20190612.000014') AO5\\r\\\\s('AO6.SA03008L.20190612.000014') AO6\\r\\\\s('AO7.SA03008L.20190612.000014') AO7\\r\\\\s('AO8.SA03008L.20190612.000014') AO8\"\nX ModifyGraph mirror(bottom)=1\nX ModifyGraph width=216\nX ModifyGraph height={Aspect,0.6}\nX ModifyGraph Log(bottom)=0\nX ModifyGraph Log(left)=0\nX \n", 15 "E index vs Field":cluster{i32[], dbl[]}(graph))   [LabVIEW 2016]
uses:
  <vilib>/Utility/miscctls.llb/LVOffsetAndMultiplierTypeDef.ctl
  <vilib>/Analysis/3filter.llb/Savitzky-Golay Filter (DBL).vi
  <vilib>/Analysis/2dsp.llb/Decimate (single shot, DBL).vi
  <userlib>/LevyLab/LV to ITX/LVtoITX.lvclass
  <vilib>/Analysis/NI_AALPro.lvlib
  <vilib>/Analysis/NI_AALBase.lvlib
panel:
  in  "VRM mode":bool
  in  "Ring":u16(ring) items=["default", "DIFF"]
  in  "decimating factor":i32=1
  in  "decimate files":i32=1
  in  "side points":i32=6
  in  "fit points":dbl=10.0
  in  "dy/dx vs x":bool=TRUE
  in  "Portion of data":cluster{dbl, dbl}(slide)={0.75, 0.25} scale=0.0..1.0
  in  "length 2":i32=1000000
  in  "index 2":i32
  out "Ns":T1(array[cluster])=[{"N1"=0.0, "N2"=0.0, "N3"=0.0, "N4"=0.042391166609344784}]
  in  "SE?":bool
  in  "D  is time?":bool
  in  "B is time?":bool
  out "time":string[][](table)=[["6/13/2019", "4:54 PM"]]
  in  "Use Folder Index File?":bool
  in  "Generate Folder Index File?":bool
  in  "Ez name":string="Conductance (S)"
  in  "Ey name":string="BY (T)"
  in  "Ex name":string="Vsg (mV)"
  in  "C y name":string="voltage"
  in  "D x name":string="Vsg"
  in  "A y name":string="current"
  in  "B x name":string="Vsg"
  in  "recolor traces?":bool
  in  "Ex":T3={"Offset"=0.0, "Multiplier"=1.0}
  in  "Ey":T3={"Offset"=0.0, "Multiplier"=1.0}
  out "Path":path=path "G:/My Drive/ansom/Data/PPMS2/SA03008L.20190612/030_phi_90_Vamp_bg=30_IV_Testing/SA03008L.20190612.000014.itx"
  out "counter":i32
  in  "pattern":string="*.itx"
  # "A1-A2\nC1-C2\nE-E2"
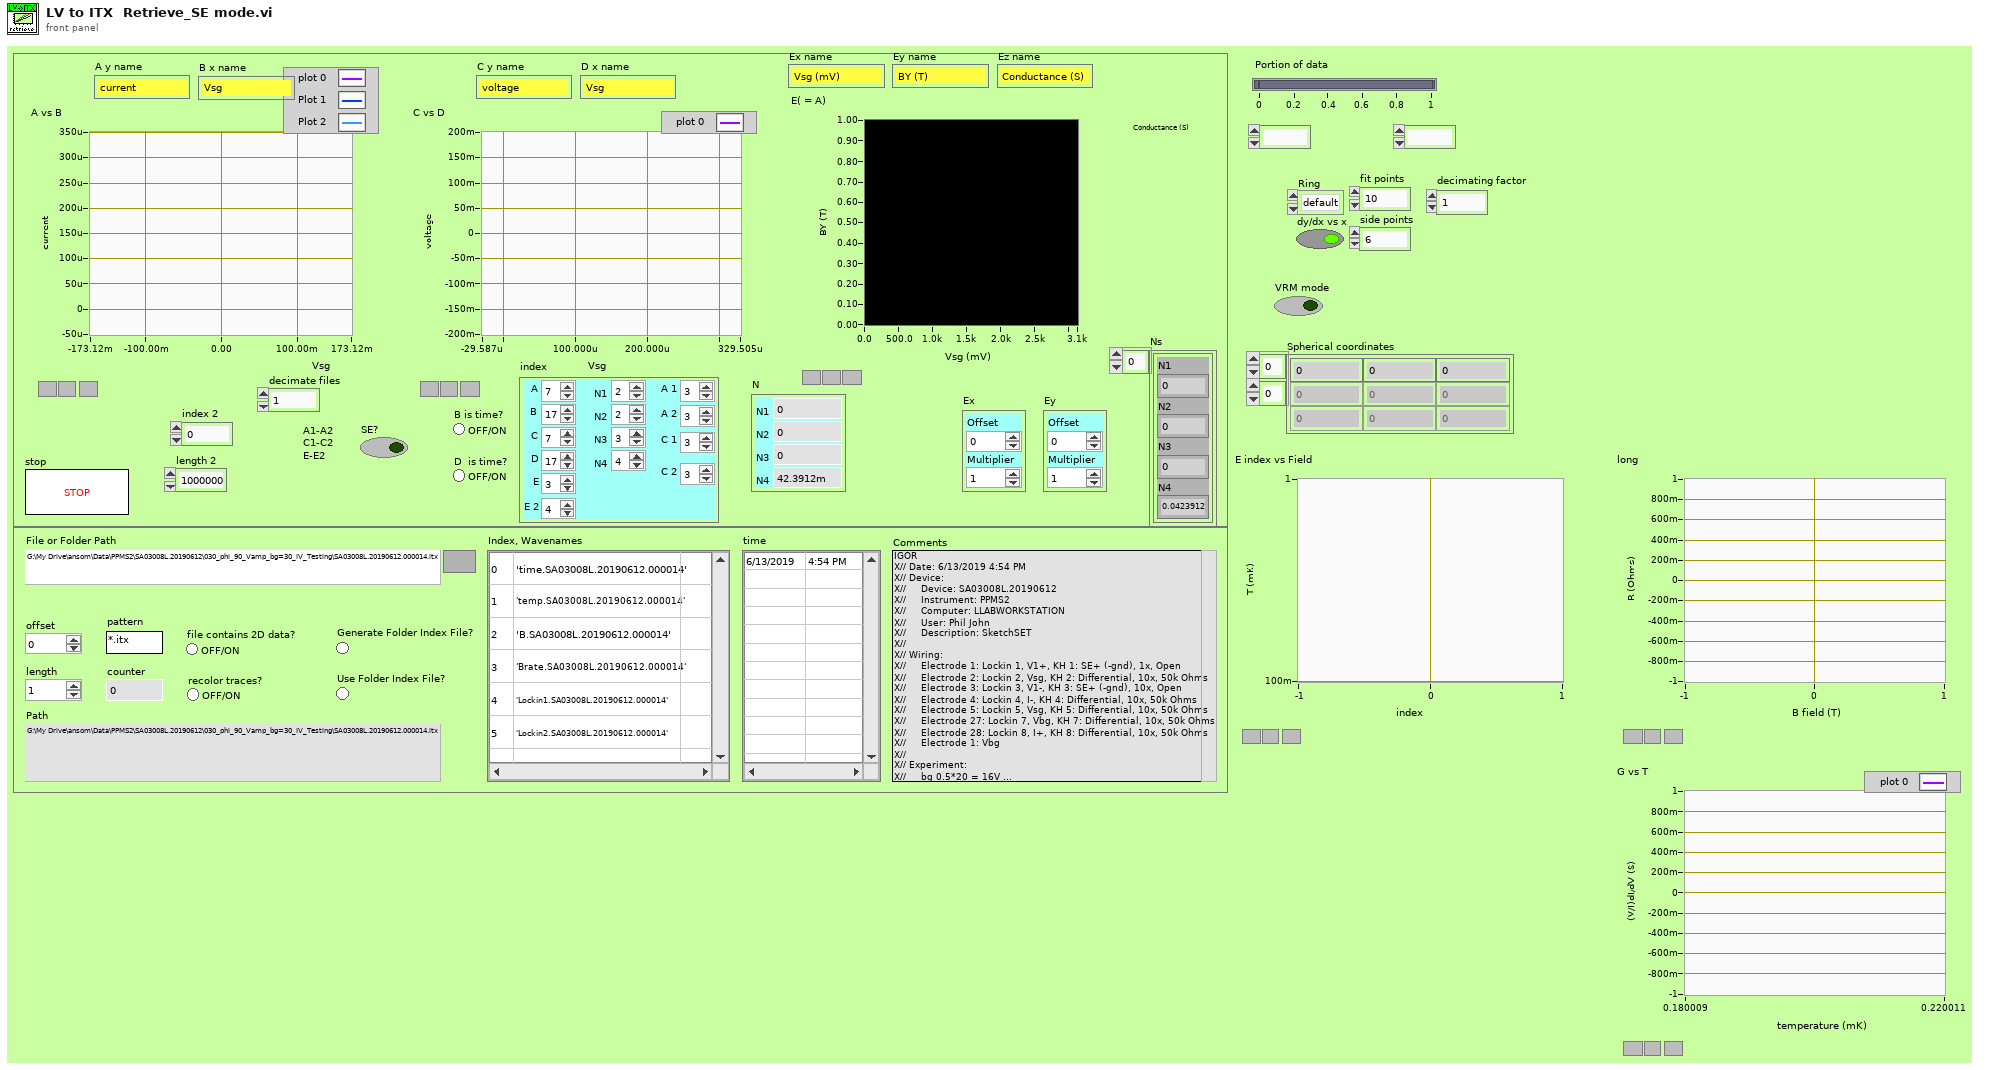
[diagram p1: front panel]
types:
  T1 = cluster{"N1":dbl, "N2":dbl, "N3":dbl, "N4":dbl}[]
  T2 = cluster{"A":i32, "B":i32, "C":i32, "D":i32, "E":i32, "N1":i32, "N2":i32, "N3":i32, "N4":i32, "A 1":i32, "A 2":i32, "C 1":i32, "C 2":i32, "E 2":i32}
  T3 = typedef "LVOffsetAndMultiplierTypeDef.ctl" = cluster{"Offset":dbl, "Multiplier":dbl}
  T4 = cluster{"Decimated Array":dbl[], "Decimated Array":dbl[]}
  T5 = cluster{"Decimated Array":dbl[], "Filtered X":dbl[]}
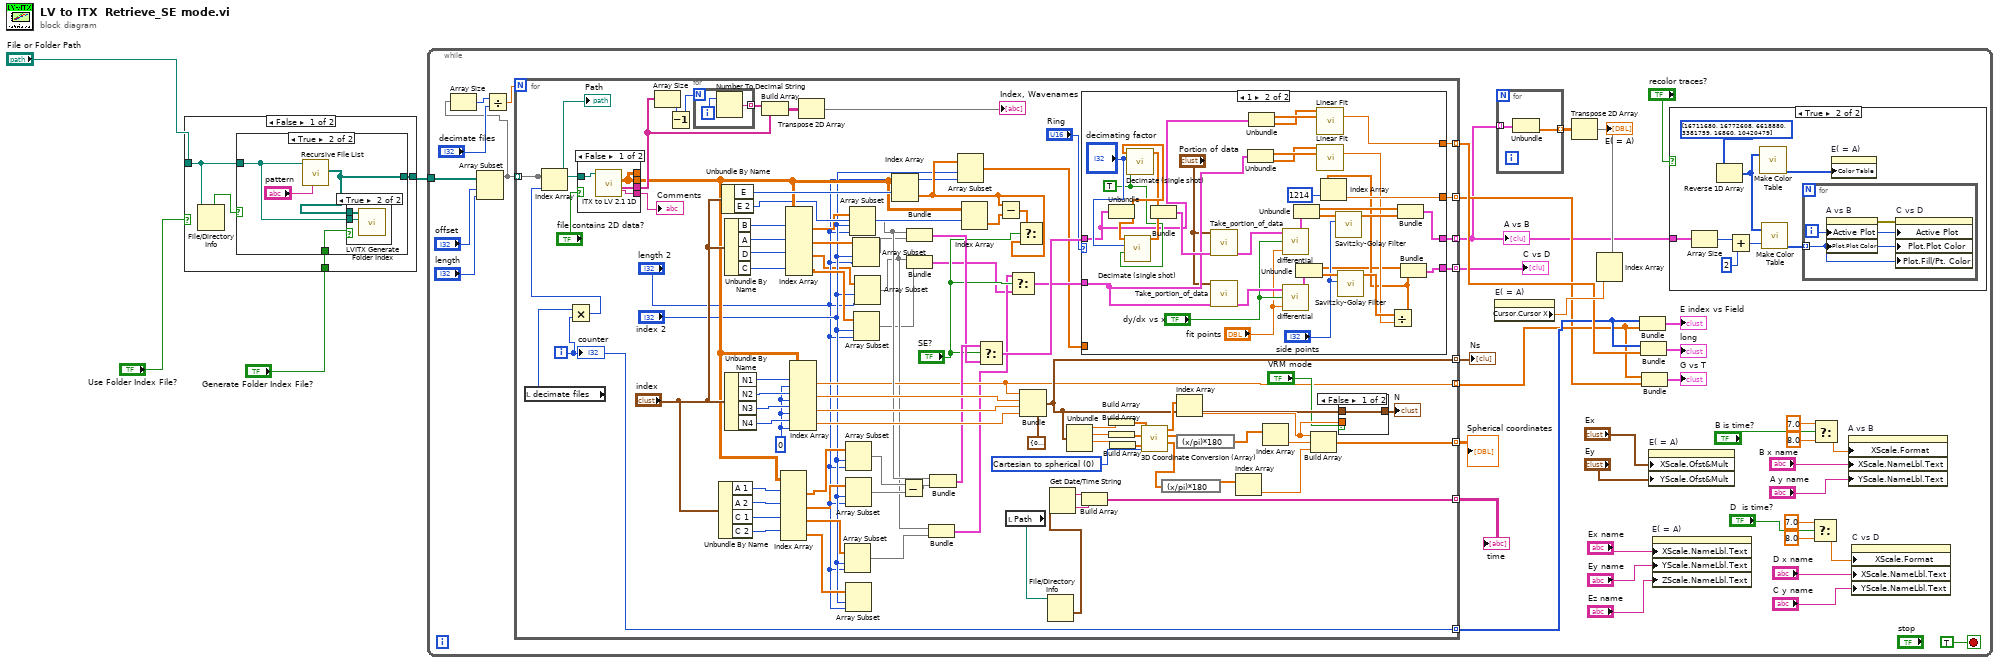
[diagram p0: block diagram]
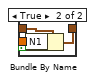
[diagram p3: hidden frame]
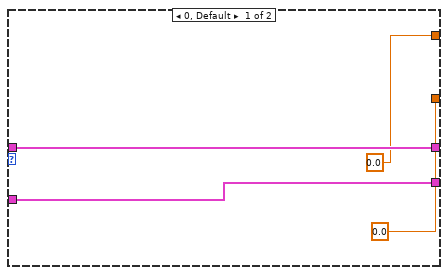
[diagram p4: hidden frame]
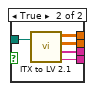
[diagram p5: hidden frame]
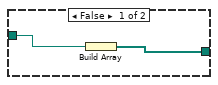
[diagram p6: hidden frame]
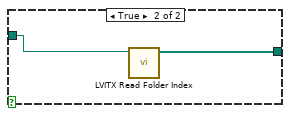
[diagram p8: hidden frame]
diagram:
  n1 = case shown="False" "Use Folder Index File?" {
    tunnel: [w6 w17] -> w2
    tunnel: "File or Folder Path" -> [w8 w18]
    tunnel: "Generate Folder Index File?" -> [w5 _]
    frame False {
      n2 = File/Directory Info(path=w8) -> (directory=w7:bool)  [unwired: 1 in, 6 out]
      n3 = case shown="True" w7 {
        tunnel: [w10 w13] -> w6
        tunnel: w8 -> [w9 w12]
        tunnel: w5 -> [_ w11]
        frame False {
          n4 = Build Array(w9) -> (w10:path[])
        }
        frame True {
          n5 = call <vilib>:"Recursive File List.vi"("pattern"="pattern", "Folder Path"=w12) -> ("All Files in Dir"=w13:path[])  [unwired: 5 in, 4 out]
          n6 = case shown="True" w11 {
            tunnel: w13 -> [_ w16]
            tunnel: w12 -> [_ w15]
            frame False {
            }
            frame True {
              n7 = call <userlib>:"LVITX Generate Folder Index.vi"("File or Folder Path"=w15, "All Files in Dir"=w16) -> ()  [unwired: 10 in]
            }
          }
        }
      }
    }
    frame True {
      n8 = call <userlib>:"LVITX Read Folder Index.vi"("File or Folder Path"=w18) -> ("Array"=w17:path[])  [unwired: 10 in]
    }
  }
  n9 = while {
    tunnel: w2 -> [w36]
    stop <- TRUE stop-if-true
    n10 = Array Subset(array=w36, index="offset", length="length") -> (w32:path[])
    n11 = Array Size(array=w32) -> (size(s)=w35:i32)
    n12 = Divide(x=w35, y="decimate files") -> (x/y=w33:dbl)
    n13 = for {
      N: w33 -> [_]
      tunnel: w32 -> [w164]
      tunnel: [w164] -> _ mode=indexing
      tunnel: [w99] -> w19 mode=indexing
      tunnel: [w98] -> w20 mode=indexing
      tunnel: [w139] -> w50 mode=indexing
      tunnel: [w87] -> w39 mode=indexing
      tunnel: [w97] -> w37 mode=indexing
      tunnel: [w91] -> w29 mode=indexing
      tunnel: [w90] -> w21 mode=indexing
      tunnel: [w84] -> w25 mode=indexing
      tunnel: [w83] -> w24 mode=indexing
      i -> [w84]
      w114 = u16 0 items=["Cartesian to spherical", "spherical to Cartesian", "Cartesian to cylindrical", "cylindrical to Cartesian", "spherical to cylindrical", "cylindrical to spherical"] ("conversion type")
      w137 = 0 ("disabled index (col)")
      n14 = local read "decimate files"() -> (w94:i32)
      n15 = Multiply(x=w94, y=w84) -> (x*y=w95:i32)
      n16 = Index Array(array=w164, index=w95) -> (element=w96:path)
      "Path" <- w96
      n17 = case shown="False" "file contains 2D data?" {
        tunnel: [w213 w216] -> w165
        tunnel: [w211 w217] -> w128
        tunnel: w96 -> [w212 w218]
        tunnel: [w210 w215] -> w157
        tunnel: [w211 w214] -> _
        frame False {
          n18 = call <userlib>:"ITX to LV 2.1 1D.vi"("file (use dialog)"=w212) -> ("wave names"=w210:string[], "1D arrays"=w211:dbl[][], "Notes"=w213:string)  [unwired: 6 in, 2 out]
        }
        frame True {
          n19 = call <userlib>:"ITX to LV 2.1.vi"("file (use dialog)"=w218) -> ("2D array"=w214:dbl[][], "1D arrays"=w217:dbl[][], "wave names"=w215:string[], "Notes"=w216:string)  [unwired: 1 in]
        }
      }
      "Comments" <- w165
      n20 = Array Size(array=w157) -> (size(s)=w160:i32)
      n21 = Decrement(x=w160) -> (x-1=w159:i32)
      n22 = for {
        N: w159 -> [_]
        tunnel: [w208] -> w162 mode=indexing
        i -> [w209]
        n23 = Number To Decimal String(number=w209) -> (decimal integer string=w208:string)  [unwired: 1 in]
      }
      n24 = Unbundle By Name("index") -> ("A 1"=w136:i32, "A 2"=w135:i32, "C 1"=w134:i32, "C 2"=w133:i32)
      n25 = Unbundle By Name("index") -> ("E"=w150:i32, "E 2"=w127:i32)
      n26 = Unbundle By Name("index") -> ("B"=w149:i32, "A"=w148:i32, "D"=w147:i32, "C"=w146:i32)
      n27 = Unbundle By Name("index") -> ("N1"=w151:i32, "N2"=w152:i32, "N3"=w153:i32, "N4"=w154:i32)
      n28 = Build Array(w162, w157) -> (w158:string[][])
      n29 = Index Array(array=w128, index (row) #1=w136, index (row) #2=w135, index (row) #3=w134, index (row) #4=w133) -> (element #1=w119:dbl[], element #2=w117:dbl[], element #3=w116:dbl[], element #4=w115:dbl[])  [unwired: 4 in]
      n30 = Index Array(array=w128, index (row) #1=w149, index (row) #2=w148, index (row) #3=w147, index (row) #4=w146) -> (element #1=w124:dbl[], element #2=w122:dbl[], element #3=w74:dbl[], element #4=w120:dbl[])  [unwired: 4 in]
      n31 = Index Array(array=w128, index (row) #1=w151, index (col) #1=w137, index (row) #2=w152, index (col) #2=w137, index (row) #3=w153, index (col) #3=w137, index (row) #4=w154, index (col) #4=w137) -> (element #1=w83:dbl, element #2=w143:dbl, element #3=w144:dbl, element #4=w156:dbl)
      n32 = Transpose 2D Array(2D array=w158) -> (transposed array=→"Index, Wavenames":string[][])
      n33 = Array Subset(array=w116, index="index 2", length="length 2") -> (w82:dbl[])
      n34 = Array Subset(array=w119, index="index 2", length="length 2") -> (w118:dbl[])
      n35 = Array Subset(array=w117, index="index 2", length="length 2") -> (w89:dbl[])
      n36 = Array Subset(array=w115, index="index 2", length="length 2") -> ()  [unwired: 1 out]
      n37 = Array Subset(array=w124, index="index 2", length="length 2") -> (w123:dbl[])
      n38 = Array Subset(array=w122, index="index 2", length="length 2") -> (w121:dbl[])
      n39 = Array Subset(array=w120, index="index 2", length="length 2") -> (w73:dbl[])
      n40 = Array Subset(array=w74, index="index 2", length="length 2") -> (w75:dbl[])
      n41 = Index Array(array=w128, index (row)=w150) -> (element=w79:dbl[])  [unwired: 1 in]
      n42 = Subtract(x=w118, y=w89) -> (x-y=w132:dbl[])
      n43 = Bundle(w123, w121) -> (w130:cluster{dbl[], dbl[]})  [unwired: 1 in]
      n44 = Bundle(w75, w73) -> (w80:cluster{dbl[], dbl[]})  [unwired: 1 in]
      n45 = Bundle(w75, w82) -> (w81:cluster{dbl[], dbl[]})  [unwired: 1 in]
      n46 = Bundle(w123, w132) -> (w131:cluster{dbl[], dbl[]})  [unwired: 1 in]
      n47 = Array Subset(array=w79, index="index 2", length="length 2") -> (w76:dbl[])
      n48 = Index Array(array=w128, index (row)=w127) -> (element=w126:dbl[])  [unwired: 1 in]
      n49 = Select(t=w131, s="SE?", f=w130) -> (s? t:f=w101:cluster{dbl[], dbl[]})
      n50 = Subtract(x=w79, y=w126) -> (x-y=w125:dbl[])
      n51 = local read "Path"() -> (w145:path)
      n52 = Select(t=w81, s="SE?", f=w80) -> (s? t:f=w100:cluster{dbl[], dbl[]})
      n53 = Select(t=w125, s="SE?", f=w79) -> ()  [unwired: 1 out]
      n54 = Bundle(cluster=cluster{"N1":dbl, "N2":dbl, "N3":dbl, "N4":dbl} {"N1"=0.0, "N2"=0.0, "N3"=0.0, "N4"=0.0}, "N1"=w83, "N2"=w143, "N3"=w144, "N4"=w156) -> (w87:cluster{"N1":dbl, "N2":dbl, "N3":dbl, "N4":dbl})
      n55 = File/Directory Info(path=w145) -> (last mod=w142:timestamp)  [unwired: 1 in, 6 out]
      n56 = Get Date/Time String(seconds (now)=w142) -> (date string=w141:string, time string=w140:string)  [unwired: 2 in]
      n57 = Unbundle(w87) -> ("N1"=w93:dbl, "N2"=w113:dbl, "N3"=w110:dbl)  [unwired: 1 out]
      n58 = case shown="1" "Ring" {
        tunnel: w101 -> [w173 w191]
        tunnel: w100 -> [w172 w180]
        tunnel: [w173 w176] -> w99
        tunnel: [w172 w175] -> w98
        tunnel: [0.0 w188] -> w91
        tunnel: [0.0 w185] -> w90
        tunnel: w76 -> [_ _]
        frame 0, Default {
        }
        frame 1 {
          w192 = TRUE ("averaging")
          n59 = Unbundle(w191) -> (w197:dbl[], w195:dbl[])
          n60 = call-poly <vilib>:"Decimate (single shot).vi"("averaging"=w192, "decimating factor"="decimating factor", "X"=w195) -> ("Decimated Array"=w194:dbl[])  [unwired: 7 in, 1 out]
          n61 = call-poly <vilib>:"Decimate (single shot).vi"("averaging"=w192, "decimating factor"="decimating factor", "X"=w197) -> ("Decimated Array"=w196:dbl[])  [unwired: 7 in, 1 out]
          n62 = Bundle("Decimated Array"=w196, "Decimated Array"=w194) -> (w198:T4)  [unwired: 1 in]
          n63 = call <userlib>:"Take_portion_of_data.vi"("input IV"=w198, "Slide"="Portion of data") -> ("Output IV"=w206:cluster{dbl[], dbl[]})  [unwired: 5 in]
          n64 = call <userlib>:"Take_portion_of_data.vi"("input IV"=w180, "Slide"="Portion of data") -> ("Output IV"=w207:cluster{dbl[], dbl[]})  [unwired: 5 in]
          n65 = Unbundle(w180) -> (w189:dbl[], w184:dbl[])
          n66 = Unbundle(w191) -> (w190:dbl[], w187:dbl[])
          n67 = call <userlib>:"differential.vi"("Numeric"="fit points", "dy/dx vs x"="dy/dx vs x", "A vs B 2"=w206) -> ("A vs B 3"=w202:T4)  [unwired: 1 in]
          n68 = call <userlib>:"differential.vi"("Numeric"="fit points", "dy/dx vs x"="dy/dx vs x", "A vs B 2"=w207) -> ("A vs B 3"=w200:T4)  [unwired: 1 in]
          n69 = Unbundle(w202) -> ("Decimated Array"=w205:dbl[], "Decimated Array"=w203:dbl[])
          n70 = Unbundle(w200) -> ("Decimated Array"=w174:dbl[], "Decimated Array"=w201:dbl[])
          n71 = call <vilib>:"Linear Fit.vi"("Y"=w187, "X"=w190) -> ("slope"=w188:dbl)  [unwired: 9 in, 4 out]
          n72 = call <vilib>:"Linear Fit.vi"("Y"=w184, "X"=w189) -> ("slope"=w182:dbl)  [unwired: 9 in, 4 out]
          n73 = call-poly <vilib>:"Savitzky-Golay Filter.vi"("side points"="side points", "X"=w203) -> ("Filtered X"=w204:dbl[])  [unwired: 8 in, 1 out]
          n74 = call-poly <vilib>:"Savitzky-Golay Filter.vi"("side points"="side points", "X"=w201) -> ("Filtered X"=w183:dbl[])  [unwired: 8 in, 1 out]
          n75 = Divide(x=w183, y=w182) -> (x/y=w181:dbl[])
          n76 = Index Array(array=w181, index=1214) -> (element=w185:dbl)
          n77 = Bundle("Decimated Array"=w205, "Filtered X"=w204) -> (w176:T5)  [unwired: 1 in]
          n78 = Bundle("Decimated Array"=w174, w181) -> (w175:cluster{"Decimated Array":dbl[], dbl[]})  [unwired: 1 in]
        }
      }
      n79 = Build Array(w141, w140) -> (w139:string[])
      n80 = Build Array(w93) -> (w112:dbl[])
      n81 = Build Array(w113) -> (w111:dbl[])
      n82 = Build Array(w110) -> (w109:dbl[])
      n83 = call <vilib>:"3D Coordinate Conversion (Array).vi"("conversion type"=w114, "Axis 3"=w109, "Axis 2"=w111, "Axis 1"=w112) -> ("Axis 3 Out"=w107:dbl[], "Axis 2 Out"=w108:dbl[], "Axis 1 Out"=w106:dbl[])  [unwired: 4 in, 1 out]
      n84 = expression code="(x/pi)*180" ("degrees to radians")(w107) -> (w104:dbl[])
      n85 = Index Array(array=w106) -> (element=w88:dbl)  [unwired: 1 in]
      n86 = expression code="(x/pi)*180" ("degrees to radians")(w108) -> (w105:dbl[])
      n87 = Index Array(array=w104) -> (element=w102:dbl)  [unwired: 1 in]
      n88 = Index Array(array=w105) -> (element=w103:dbl)  [unwired: 1 in]
      n89 = Build Array(w88, w103, w102) -> (w97:dbl[])
      n90 = case shown="False" "VRM mode" {
        tunnel: w88 -> [_ w169]
        tunnel: w87 -> [w166 w168]
        tunnel: [w166 w167] -> w86
        frame False {
        }
        frame True {
          n91 = Bundle By Name(cluster=w168, "N1"=w169) -> (w167:cluster{"N1":dbl, "N2":dbl, "N3":dbl, "N4":dbl})
        }
      }
      "N" <- w86
      "counter" <- w84
    }
    "time" <- w50
    "Ns" <- w39
    "Spherical coordinates" <- w37
    "A vs B" <- w19
    "C vs D" <- w20
    n92 = property on="E( = A)" class="IntGraph (strict)"() -> ("Cursor.Cursor X"=w30:dbl)  [unwired: 2 in, 2 out]
    n93 = for {
      tunnel: [w60] -> _ mode=indexing
      tunnel: [w61] -> w38 mode=indexing
      tunnel: w19 -> [w60] mode=indexing
      n94 = Unbundle(w60) -> ("Filtered X"=w61:dbl[])  [unwired: 1 out]
    }
    n95 = Transpose 2D Array(2D array=w38) -> (transposed array=w22:dbl[][])
    "E( = A)" <- w22
    n96 = Index Array(array=w22, index (row)=w30) -> ()  [unwired: 1 in, 1 out]
    n97 = Bundle(w25, w24) -> (→"E index vs Field":cluster{i32[], dbl[]})  [unwired: 1 in]
    n98 = Bundle(w25, w29) -> (→"long":cluster{i32[], dbl[]})  [unwired: 1 in]
    n99 = Bundle(w24, w21) -> (→"G vs T":cluster{dbl[], dbl[]})  [unwired: 1 in]
    n100 = property on="E( = A)" class="IntGraph (strict)"("XScale.Ofst&Mult"="Ex", "YScale.Ofst&Mult"="Ey") -> ()  [unwired: 2 in, 2 out]
    n101 = property on="E( = A)" class="IntGraph (strict)"("XScale.NameLbl.Text"="Ex name", "YScale.NameLbl.Text"="Ey name", "ZScale.NameLbl.Text"="Ez name") -> ()  [unwired: 2 in, 2 out]
    n102 = case shown="True" "recolor traces?" {
      tunnel: w19 -> [_ w64]
      frame False {
      }
      frame True {
        n103 = Array Size(array=w64) -> (size(s)=w65:i32)
        n104 = Reverse 1D Array(array=u32[] [16711680, 16772608, 6618880, 3381759, 16860, 10420479] ("color scale")) -> (reversed array=w63:u32[])
        n105 = Add(x=w65, y=2 ("x")) -> (x+y=w69:i32)
        n106 = call <userlib>:"Make Color Table.vi"("Array"=w63) -> ("Color Tbl"=w67:u32[])  [unwired: 1 in, 3 out]
        n107 = call <userlib>:"Make Color Table.vi"("Array"=w63, "Size"=w69) -> ("Color Tbl"=w66:u32[])  [unwired: 3 out]
        n108 = for {
          tunnel: w66 -> [w70] mode=indexing
          i -> [w71]
          n109 = property on="A vs B" class="XYGraph (strict)"("Active Plot"=w71, "Plot.Plot Color"=w70) -> (error out=w72:errorcluster)  [unwired: 2 in, 1 out]
          n110 = property on="C vs D" class="XYGraph (strict)"(error in=w72, "Active Plot"=w71, "Plot.Plot Color"=w70, "Plot.Fill/Pt. Color"=w70) -> ()  [unwired: 1 in, 2 out]
        }
        n111 = property on="E( = A)" class="IntGraph (strict)"("Color Table"=w67) -> ()  [unwired: 2 in, 2 out]
      }
    }
    n112 = Select(t=7.0, s="D  is time?", f=8.0) -> (s? t:f=w44:dbl)
    n113 = Select(t=7.0, s="B is time?", f=8.0) -> (s? t:f=w45:dbl)
    n114 = property on="A vs B" class="XYGraph (strict)"("XScale.Format"=w45, "XScale.NameLbl.Text"="B x name", "YScale.NameLbl.Text"="A y name") -> ()  [unwired: 2 in, 2 out]
    n115 = property on="C vs D" class="XYGraph (strict)"("XScale.Format"=w44, "XScale.NameLbl.Text"="D x name", "YScale.NameLbl.Text"="C y name") -> ()  [unwired: 2 in, 2 out]
  }
